vi "simulated image deformation.vi"(9 "Stop":bool, 11 "file path (use dialog)":path=path "F:/20240411-145056tdTomato zfluctuate dark small/20240411-145056tdTomato zfluctuate dark small.3DU16") -> ()   [LabVIEW 2024]
doc: "This example shows how to use the color pattern matching tools in NI Vision.\n\nYou use color pattern matching to locate known reference or fiducial patterns in an image quickly. Pattern matching is the key to many applications. Color pattern matching can provide your application with information about the presence or absence, number, and location of the model within an image.\n\nYou use color pattern matching in the following three general applications areas:\n\n* Alignment -- Determine the position and orientation of a known object by locating features. You use the features as points of reference on the object.\n\n* Gauging -- Measure lengths, diameters, angles, and other critical dimensions. If the measurements fall outside of set tolerance levels, the component is rejected. You sometimes use gauging in-line with the manufacturing process and off-line. If you make the measurements off-line, a sample of components is used to determine the quality of a lot or batch of manufactured components.\n\n* Inspection -- Detect simple flaws, such as missing parts or unreadable printing."
uses:
  <vilib>/gmath/NumericalOptimization/stopping criteria.ctl
  <vilib>/Analysis/baseanly.llb/Real A x B.vi
  <vilib>/Analysis/baseanly.llb/A x Vector.vi
  <vilib>/gmath/NumericalOptimization/Downhill Simplex.vi
  <vilib>/vision/NI_Vision_Development_Module.lvlib
  <vilib>/gmath/NI_Gmath.lvlib
  <vilib>/Analysis/NI_AALBase.lvlib
panel:
  in  "save transformed imgs":bool=TRUE
  out "A x B":dbl[][][](array[numeric])=[[[1.0252319039814008, 0.002391061207094415, -0.3573751785157772], [0.00737380006384733, 1.023351696337477, -5.931741689900512], [4.801742722373331e-05, -1.5076143397823732e-05, 1.0]], [[1.032657460981609, -0.004112535189805674, 0.9921109023203691], [0.014233192177529825, 1.0208690943004752, -7.9981262414118754], [7.030577164981777e-05, -4.3262018120171305e-05, 1.0001558400761408]], [[1.0416733185763245, 0.006155557532026288, -2.0796096172703544], [0.015025223132497195, 1.0275947891361181, -7.698789210595932], [9.848724819265994e-05, -4.749138408643344e-05, 1.0002152245800837]], [[1.055582542463075, 0.0225232241207663, -6.272162520913962], [0.015671378565617424, 1.0390878659055158, -6.578682702191399], [0.00011065087078061124, -1.1644079672646958e-05, 0.9999239310237085]], [[1.0696837271299575, 0.0504127718928557, -10.16158458953805], [0.016405251487257792, 1.0626775335818377, -6.853459701654355], [0.00012715279311096902, 5.854990616084134e-05, 0.9993898132887179]], [[1.0867852876742778, 0.05466443617762524, -10.645243835104656], [0.0215449194026129, 1.0885495889388574, -10.976399560961317], [0.00016645941245247426, 6.81093126769533e-05, 0.9989678064999458]], [[1.1109676198793976, 0.055385921129969956, -11.411221140746001], [0.02718487606984163, 1.1036287605452453, -13.550538925915514], [0.00021282122893302702, 6.923321844189429e-05, 0.9985256438980302]], [[1.1111042461542384, 0.050999241521229886, -10.754894691290525], [0.02730121211520052, 1.093865956251593, -12.65523517648029], [0.00022306723318648547, 3.6131640344551076e-05, 0.9988250940132484]], [[1.1118110959717575, 0.05618805365262508, -11.553002851896442], [0.027990916395066647, 1.0954167080541724, -11.28573727695852], [0.0002295058388808017, 4.6619913963022765e-05, 0.998647179090953]], [[1.1261894436159139, 0.09733031423529623, -19.260741205606603], [0.029220748081624653, 1.1165854803933235, -11.610522949858835], [0.00025346518882477767, 9.924433055073616e-05, 0.9978814999070178]]]
  out "Intensity Graph 7":dbl[][](graph)
  out "Intensity Graph 3":u16[][](graph)
  in  "z index":i32=48
  in  "quit review":bool
  in  "review index":i32=700
  out "Intensity Graph 2":u16[][](graph)
  out "Waveform Graph":dbl[][](graph)=[[0.0, -0.08806760786646446, -0.16032994108789017, -0.2183501586951051, -0.26369141971893734, -0.2979168831902148, -0.3225897081397656, -0.33927305359841764, -0.3495300785969989, -0.35492394216633755, -0.35701780333726146, -0.3573748211405988, -0.3328497292755918, -0.25364666922385326, -0.13116245216132086, 0.022798969999970276, 0.19643364534798619, 0.37793762197069186, 0.5555069479560524, 0.7173376713920336, 0.8516258403666004, 0.9465675029677187, 0.9903587072833533, 0.9650749491075363, 0.8574975473775769, 0.6782939355281823, 0.43882181480620885, 0.15043888645851322, -0.17549714826804919, -0.527628588126619, -0.8945977318703406, -1.2650468782523596, -1.6276183260258152, -1.9709543739438526, -2.296946156935724, -2.640927730904358, -3.0025556475511013, -3.3783195711163714, -3.7647091658405802, -4.158214095964146, -4.555324025727483, -4.952528619371011, -5.346317541135141, -5.733180455260291, -6.109607025986877, -6.48106926036093, -6.883860677888618, -7.311417492005393, -7.751127569084709, -8.190378775500008, -8.616558977624749, -9.017056041832381, -9.379257834496357, -9.690552221990131, -9.938327070687153, -10.109970246960875, -10.201151879841863, -10.267024567986702, -10.321911211707524, -10.367952569544704, -10.407289400038614, -10.44206246172963, -10.474412513158125, -10.506480312864474, -10.540406619389051, -10.57833219127223, -10.622397787054384, -10.675173119096588, -10.742515845409994, -10.822471601698131, -10.910905333332167, -11.003681985683269, -11.096666504122606, -11.185723834021344, -11.266718920750652, -11.335516709681697, -11.387982146185648, -11.419980175633668, -11.427288124583471, -11.405851457892762, -11.359375623120723, -11.293638889824585, -11.21441952756158, -11.127495805888934, -11.038645994363877, -10.953648362543642, -10.878281179985455, -10.818322716246547, -10.779551240884148, -10.767640545611597, -10.776910242635998, -10.800863446106137, -10.838842296024412, -10.89018893239322, -10.954245495214964, -11.030354124492039, -11.117856960226845], [0.0, -0.6990844119063075, -1.377904026033752, -2.0323701215933294, -2.658393977796034, -3.251886873852863, -3.808760088974812, -4.324924902372875, -4.79629259325805, -5.21877444084133, -5.588281724333714, -5.900725722946196, -6.176724297406029, -6.449291732458249, -6.714149880756897, -6.9666333680901396, -7.202076820246148, -7.415814863013091, -7.603182122179137, -7.759513223532458, -7.880142792861221, -7.960405455953598, -7.995635838597756, -7.9948336322923925, -7.986480781535741, -7.972204257323417, -7.952558476324648, -7.928097855208662, -7.899376810644687, -7.86694975930195, -7.83137111784968, -7.793195302957104, -7.75297673129345, -7.711269819527946, -7.660478807106392, -7.5779837528866185, -7.469326611741255, -7.342219431575375, -7.2043742602940535, -7.0635031458023665, -6.927318136005389, -6.803531278808196, -6.699854622115862, -6.624000213833463, -6.583680101866072, -6.579962872361264, -6.585233956995526, -6.595346634978383, -6.610147040936223, -6.629481309495433, -6.6531955752824, -6.681135972923512, -6.713148637045156, -6.749079702273719, -6.788775303235589, -6.832081574557153, -6.891291945954723, -7.053502480097667, -7.3192333957798015, -7.668537856253234, -8.081469024770076, -8.538080064582442, -9.01842413894243, -9.502554411102155, -9.970524044313727, -10.402386201829254, -10.778194046900845, -11.084284209007102, -11.385729309992561, -11.698136370665495, -12.012812146340236, -12.32106339233112, -12.614196863952477, -12.883519316518646, -13.120337505343956, -13.31595818574274, -13.46168811302933, -13.548834042518063, -13.569906497288047, -13.551957342469379, -13.51166631084667, -13.452158545978971, -13.376559191425343, -13.287993390744841, -13.18958628749652, -13.084463025239433, -12.975748747532641, -12.866568597935194, -12.760047720006153, -12.659065885842333, -12.543790814013336, -12.40520389539235, -12.250530202818402, -12.086994809130518, -11.921822787167729, -11.762239209769062, -11.61546914977354], [498.0, 498.05959291224764, 498.1109505097321, 498.1546182800102, 498.19114171063876, 498.22106628917453, 498.2449375031743, 498.2633008401948, 498.27670178779294, 498.2856858335255, 498.2907984649492, 498.29258516962085, 498.28854436784206, 498.27453904241014, 498.2509591731421, 498.2182421278122, 498.1768252741945, 498.1271459800634, 498.0696416131931, 498.00474954135774, 497.93290713233154, 497.85455175388876, 497.7701207738036, 497.61713712408425, 497.2777173834449, 496.78789154147364, 496.1891634558678, 495.52303698432473, 494.8310159845418, 494.1546043142164, 493.53530583104583, 493.01462439272746, 492.6340638569586, 492.4351280814367, 492.4055259436575, 492.392373253152, 492.38226987404346, 492.3744822410049, 492.3682767887094, 492.3629199518301, 492.3576781650401, 492.3518178630124, 492.34460548042017, 492.3353074519365, 492.3231902122344, 492.30650694071056, 492.28031112090554, 492.2448781840679, 492.2011884696724, 492.1502223171939, 492.0929600661073, 492.0303820558875, 491.9634686260093, 491.8932001159475, 491.820556865177, 491.74651921317275, 491.66865653803535, 491.5644471740417, 491.43579776771617, 491.29028385163474, 491.1354809583733, 490.9789646205077, 490.82831037061396, 490.69109374126793, 490.57489026504555, 490.4872754745227, 490.4358249022752, 490.4257655490913, 490.43149698256036, 490.44293482140483, 490.458727548562, 490.4775236469694, 490.49797159956444, 490.51871988928445, 490.5384169990669, 490.5557114118492, 490.56925161056876, 490.577686078163, 490.57847624470804, 490.5401514953157, 490.4548658284808, 490.33021692570134, 490.1738024684751, 489.99322013829993, 489.7960676166738, 489.5899425850944, 489.38244272505966, 489.18116571806746, 488.99370924561566, 488.8275830414089, 488.67949517238, 488.54146103744847, 488.4096151399728, 488.2800919833113, 488.14902607082234, 488.01255190586426, 487.8668039917954], [0.0, -0.34659355840331935, -0.6697552209281179, -0.967562437605149, -1.2380926584651664, -1.4794233335389235, -1.689631912857174, -1.8667958464506709, -2.0089925843501684, -2.1142995765864194, -2.1807942731901786, -2.2065541241921984, -2.187944773997436, -2.1261760296745087, -2.0289093348903626, -1.9038526962348445, -1.7587141202978014, -1.6012016136690805, -1.439023182938529, -1.2798868346959935, -1.1315005755313214, -1.0015724120343592, -0.8978103507949546, -0.8196809058998543, -0.7514634450780548, -0.690599285840092, -0.6351229030496413, -0.5830687715703788, -0.5324713662659806, -0.4813651620001232, -0.4277846336364825, -0.3697642560387343, -0.3053385040705554, -0.23254185259562143, -0.14456043497485793, -0.027999389199703073, 0.11114401645705166, 0.2654873174264595, 0.42764804913957155, 0.590243747027441, 0.7458919465211207, 0.8872101830516632, 1.0068159920501203, 1.097326908947545, 1.1513604691749901, 1.1688676165503586, 1.180922417594905, 1.191940545301066, 1.2018861553343343, 1.210723403360202, 1.2184164450441612, 1.224929436051705, 1.230226532048325, 1.2342718886995137, 1.2370296616707637, 1.2384640066275672, 1.231821935776551, 1.170744324711977, 1.0569070651791723, 0.9031435851839223, 0.7222873127320133, 0.5271716758292289, 0.33063010248135905, 0.14549602069418777, -0.015397141526498848, -0.1392159561749151, -0.213126995245275, -0.22806519538413308, -0.22410185444698455, -0.2157144573525903, -0.20328602675556465, -0.187199585310522, -0.16783815567207672, -0.1455847604948432, -0.12082242243343559, -0.09393416414246869, -0.06530300827655669, -0.03531197749031392, -0.004049634139276918, 0.0359271098690905, 0.0871275237671033, 0.14837358367929487, 0.21848726573019667, 0.2962905460443419, 0.3806054007462635, 0.47025380596049393, 0.5640577378115662, 0.6608391724240136, 0.7594200859223673, 0.8588240958035979, 0.976263368252154, 1.1185316498879931, 1.2787694647325516, 1.4501173368072657, 1.625715790133572, 1.798705348732907, 1.96222653662671], [498.0, 498.352995504663, 498.6963739058205, 499.0290531199109, 499.3499510633724, 499.65798565264345, 499.9520748041623, 500.23113643436733, 500.49408845969685, 500.7398487965893, 500.96733536148287, 501.17546607081596, 501.37464179085134, 501.5789093950214, 501.7835485008412, 501.98365143314686, 502.1743105167747, 502.35061807656086, 502.50766643734164, 502.6405479239532, 502.74435486123184, 502.81417957401374, 502.8451143871352, 502.82378743572696, 502.7356884268529, 502.5925893443046, 502.4070972806018, 502.1918193282643, 501.9593625798119, 501.7223341277643, 501.49334106464136, 501.2849904829628, 501.10988947524845, 500.98064513401806, 500.8987728782318, 500.8335975692704, 500.77961668207456, 500.7338112382921, 500.6931622595708, 500.65465076755834, 500.6152577839025, 500.5719643302511, 500.5217514282519, 500.4616000995526, 500.38849136580103, 500.2921931047241, 500.1402738909532, 499.93828511817765, 499.69684350399683, 499.42656576601024, 499.13806862181735, 498.84196878901764, 498.5488829852105, 498.2694279279956, 498.01422033497215, 497.7938769237398, 497.61279826542494, 497.4325400401901, 497.24841032488905, 497.06512645930275, 496.887405783212, 496.7199656363976, 496.56752335864036, 496.43479628972113, 496.32650176942064, 496.2473571375198, 496.20207973379945, 496.19311773343514, 496.1942811140667, 496.19680986244845, 496.2006685681868, 496.20582182088845, 496.2122342101597, 496.2198703256072, 496.2286947568374, 496.2386720934568, 496.2497669250719, 496.2619438412893, 496.27675996106404, 496.3345542190964, 496.4438852365347, 496.5925793326237, 496.76846282660824, 496.9593620377332, 497.15310328524333, 497.33751288838346, 497.50041716639845, 497.62964243853304, 497.71301502403213, 497.73842217131727, 497.70385651449106, 497.61900493959655, 497.49237882358017, 497.3324895433883, 497.1478484759674, 496.9469669982638, 496.738356487224], [299.0, 298.8687898245559, 298.74114208501135, 298.61822224462526, 298.5011957666566, 298.3912281143645, 298.2894847510077, 298.19713113984534, 298.11533274413637, 298.0452550271398, 297.98806345211443, 297.94492348231944, 297.9134972964784, 297.88817502359996, 297.86760770201903, 297.85049603737355, 297.8355407353016, 297.82144250144114, 297.80690204143025, 297.7906200609068, 297.77129726550896, 297.7476343608746, 297.7183320526418, 297.6729729654948, 297.5946975659272, 297.49035444654606, 297.3676103274553, 297.23413192875864, 297.0975859705601, 296.9656391729634, 296.84595825607255, 296.74620993999133, 296.6740609448236, 296.6371779906733, 296.63285238579186, 296.6314376949938, 296.6303894838692, 296.6296134483004, 296.6290152841698, 296.6285006873597, 296.6279753537525, 296.6273449792306, 296.62651525967635, 296.6253918909721, 296.62388056900016, 296.6140899421671, 296.5617806883245, 296.47048352115365, 296.3490125456797, 296.20618186692786, 296.0508055899233, 295.8916978196913, 295.7376726612569, 295.5975442196455, 295.4801265998821, 295.3942339069921, 295.3449895176176, 295.3096259667366, 295.28117834008566, 295.2579055224981, 295.23806639880723, 295.21991985384636, 295.20172477244876, 295.18174003944773, 295.15822453967667, 295.12943715796877, 295.0936367791574, 295.04652465511975, 294.9565215236572, 294.82231536714386, 294.6536774701274, 294.4603791171553, 294.2521915927753, 294.0388861815351, 293.8302341679821, 293.6360068366641, 293.4659754721286, 293.32991135892325, 293.2363100581014, 293.15805098242436, 293.0815909138026, 293.0081523302429, 292.9389577097521, 292.8752295303369, 292.81819027000427, 292.76906240676084, 292.72906841861345, 292.69943078356897, 292.6813719796341, 292.6761269685125, 292.6852826941717, 292.70728856110696, 292.7392532875312, 292.77828559165727, 292.8214941916981, 292.8659878058665, 292.9088751523754], [0.0, 0.07070781292600659, 0.13222535643952152, 0.18507884903170793, 0.22979450919372876, 0.2668985554167473, 0.2969172061919265, 0.32037668001042946, 0.33780319536341913, 0.3497229707420588, 0.3566622246375115, 0.35914717554094033, 0.3482915577971586, 0.3131532160574969, 0.2588059350305878, 0.19048024915228876, 0.11340669285845648, 0.03281580058494821, -0.04606189323237858, -0.11799585415766728, -0.1777555477550603, -0.22011043958870102, -0.23982999522273174, -0.24086489926704457, -0.24116329701618808, -0.2414315752675673, -0.24166968279406276, -0.241877568368555, -0.24205518076392457, -0.24220246875305196, -0.24231938110881773, -0.2424058666041024, -0.2424618740117865, -0.24248735210475061, -0.23928013016051664, -0.22283171328184445, -0.19318622311013947, -0.15120424894823825, -0.0977463800989781, -0.03367320586519559, 0.0401546844502724, 0.12287670154458954, 0.21363225611491807, 0.3115607588584216, 0.4158016204722639, 0.5473850940108563, 0.8007768483608195, 1.1636471126890497, 1.6087885959256754, 2.10899400700081, 2.637056054844583, 3.1657674483871165, 3.6679208965585346, 4.11630910828896, 4.483724792508517, 4.7429606581473305, 4.881562758598475, 4.993013262607376, 5.098027226909434, 5.19561631939748, 5.284792207964345, 5.364566560502858, 5.433951044905852, 5.491957329066154, 5.537597080876598, 5.569881968230012, 5.587823659019229, 5.59039759879764, 5.577098493956473, 5.549774150877927, 5.510655747529718, 5.461974461879563, 5.405961471895177, 5.344847955544278, 5.280865090794581, 5.216244055613805, 5.153216027969664, 5.094012185829876, 5.040405899432335, 4.982287519870069, 4.916765597399062, 4.846611267084489, 4.774595663991526, 4.703489923185351, 4.636065179731137, 4.575092568694061, 4.5233432251393, 4.483588284132028, 4.458598880737424, 4.451115797259061, 4.460208131096691, 4.48350644105839, 4.5200988580289145, 4.569073512893016, 4.629518536535451, 4.700522059840971, 4.781172213694331], [299.0, 299.33625940798174, 299.66277170316766, 299.9749671330503, 300.2682759451221, 300.53812838687554, 300.7799547058031, 300.9891851493973, 301.16124996515055, 301.2915794005554, 301.3756037031043, 301.40875312028965, 301.4032885902406, 301.38452928812944, 301.35551881264746, 301.3190529383504, 301.27792743979387, 301.23493809153354, 301.19288066812516, 301.1545509441243, 301.12274469408663, 301.1002576925679, 301.08988571412374, 301.1191111280352, 301.23592110019075, 301.4268187584476, 301.6761400658353, 301.9682209853833, 302.28739748012123, 302.6180055130785, 302.94438104728476, 303.2508600457695, 303.5217784715623, 303.74147228769255, 303.91007911393206, 304.07017478948, 304.2246408140779, 304.3726836529518, 304.51350977132813, 304.646325634433, 304.7703377074927, 304.88475245573335, 304.9887763443812, 305.0816158386626, 305.16247740380356, 305.23059918879653, 305.28671703298335, 305.33335733023785, 305.3731385253697, 305.40867906318846, 305.44259738850366, 305.47751194612493, 305.51604118086186, 305.56080353752395, 305.61441746092095, 305.67950139586225, 305.76394374671406, 305.9055807461334, 306.10261825323084, 306.3443419748811, 306.6200376179591, 306.91899088933945, 307.23048749589714, 307.5438131445068, 307.8482535420433, 308.1330943953814, 308.3876214113959, 308.60380113913635, 308.8085558196718, 309.01059948458266, 309.20861919323085, 309.4013020049782, 309.5873349791867, 309.7654051752182, 309.9341996524345, 310.09240547019755, 310.2387096878693, 310.3717993648115, 310.4905008780819, 310.59795116076054, 310.696903954187, 310.7886709848619, 310.8745639792859, 310.9558946639597, 311.033974765384, 311.11011601005947, 311.1856301244868, 311.2618288351666, 311.3400238685996, 311.42147856390994, 311.5027067532546, 311.58148314562163, 311.6586124780547, 311.7348994875973, 311.811148911293, 311.8881654861853, 311.9667539493179]]
  in  "stop":bool
  in  "skip matching":bool
  out "size(s)":i32[](array[numeric])=[159, 184]
  out "transform index":i32=998
  out "error out 2":errorcluster
  out "error out":errorcluster
  in  "mabiki":i32=10
  out "appended array 3":i32[](array[numeric])=[184, 159]
  out "minimum 2":dbl[](array[numeric])=[49.34280549447182, 30.507003653054642, 447.31274204038084, 30.457516913102424, 447.59510849908503, 269.39846570126116, 53.656175912030534, 269.1288380732932]
  out "appended array 2":sgl[](array[numeric])
  out "appended array":dbl[](array[numeric])=[50.0, 30.0, 449.0, 270.0]
  out "Numeric":i32=9993
  out "num of volumes":i32=9995
  out "sqrt(x) 4":dbl=2040.3038989327056
  out "sqrt(x) 3":dbl
  out "sqrt(x) 2":dbl=910.3411448462604
  out "sqrt(x)":dbl=891.563233876319
  out "max value 2":dbl=16649.0
  out "max value":dbl=16161.0
  out "minimum":dbl[](array[numeric])=[155.64411652807632, 68.43640121785279, 338.3202861949042, 68.35157731671751, 340.3174931085275, 225.28530291703504, 161.01996406448592, 233.55726960411664]
  out "number of function evaluations":i32=252
  out "f(minimum)":dbl=794885.0 format="%#_6f"
  out "Global Rectangle":i32[](array[numeric])=[156, 71, 340, 230]
  out "Intensity Graph 6":i16[][](graph)
  in  "stopping criteria":T1={"function tolerance"=100.0, "parameter tolerance"=0.0001, "max iterations"=2000, "max function calls"=100000, "gradient tolerance"=1e-06, "max time (sec)"=-1.0}
  in  "y":i32=5
  in  "max 3":dbl=100.0
  out "Intensity Graph 5":i16[][](graph)
  out "Matches (pixel)":T2(array[cluster])=[{"Position"={"x"=247.77678, "y"=146.75125}, "Angle"=0.9103387, "Scale"=1.0, "Score"=963.9151, "Bounding Box"=[{"x"=155.0332, "y"=69.21496}, {"x"=338.0101, "y"=66.30749}, {"x"=340.52036, "y"=224.28754}, {"x"=157.54346, "y"=227.195}, {"x"=155.0332, "y"=69.21496}]}] {"Bounding Box"."y" format="%.2f"; "Bounding Box"."x" format="%.2f"; "Score" format="%.2f"; "Scale" format="%.2f"; "Angle" format="%.2f"; "Position"."y" format="%.2f"; "Position"."x" format="%.2f"}
  out "ROI":T3={"Global Rectangle"=[156, 71, 340, 230], "Contours"=[{"Contour Type"=0, "ROI Type"=3, "Points"=[156, 71, 340, 230]}]}
  out "Image 2":T4(plugin-control)
  in  "z pos":i32=87
  in  "volume":i32=458
  in  "channel":i32
  in  "proj/slice":bool=TRUE
  in  "min":dbl
  in  "max":dbl=1.0
  in  "Array 2":u32[](array[colorbox])=[0, 16711680, 16776960, 16448250, 16776960, 16711680, 16448250, 16448250]
  in  "num of colors":i32=4
  in  "zoom":dbl=0.600000000000001 format="%_2g"
  out "Intensity Graph":dbl[][](graph)
  out "dimensions \n(vol, ch, z, y, x)":i32[](array[numeric])=[9995, 2, 97, 300, 499]
  out "voxel size \n(z, y, x)":dbl[](array[numeric])=[0.4095, 0.4095, 0.4095]
  out "Number of Matches":i32=1
  in  "Max # of Matches":i32=1
  in  "Minimum Score":sgl=800.0
  out "Image":T4(plugin-control)
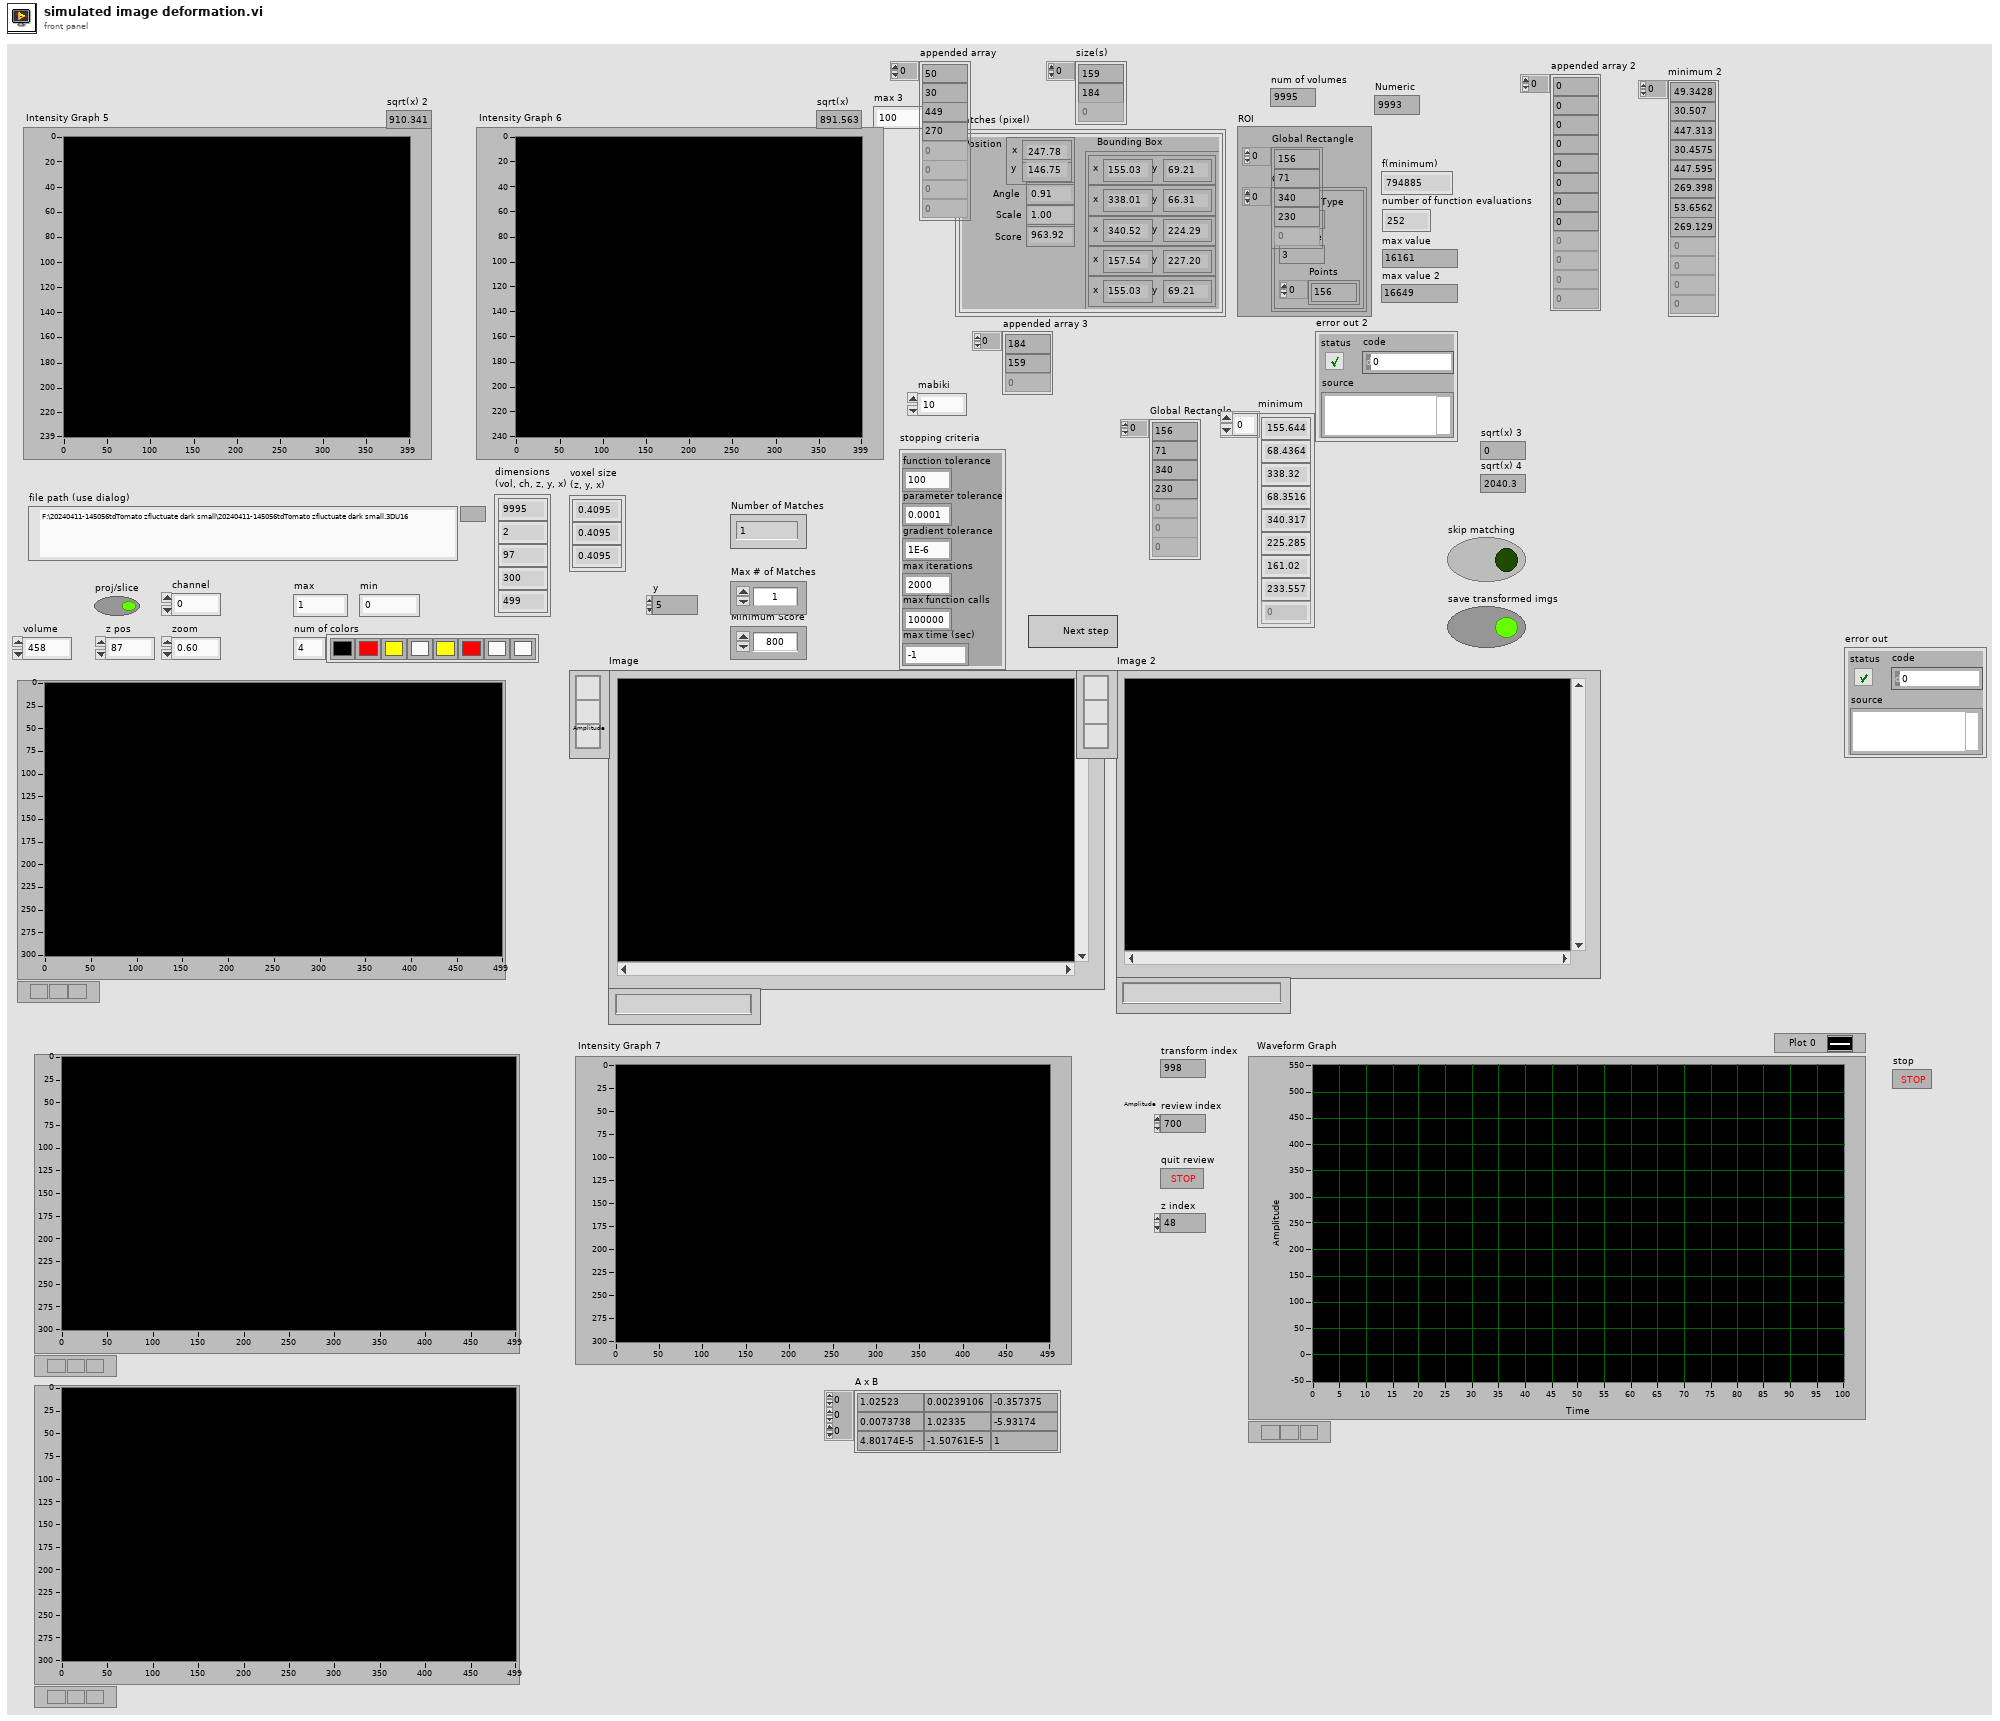
[diagram p1: front panel]
types:
  T1 = typedef "NI_Gmath.lvlib/stopping criteria.ctl" = cluster{"function tolerance":dbl, "parameter tolerance":dbl, "max iterations":i32, "max function calls":i32, "gradient tolerance":dbl, "max time (sec)":dbl}
  T2 = cluster{"Position":cluster{"x":sgl, "y":sgl}, "Angle":sgl, "Scale":sgl, "Score":sgl, "Bounding Box":cluster{"x":sgl, "y":sgl}[]}[]
  T3 = cluster{"Global Rectangle":i32[], "Contours":cluster{"Contour Type":u32, "ROI Type":u32, "Points":i32[]}[]}
  T4 = typedef "IMAQ Image.ctl" = refnum<image>
  T5 = enum16{"open", "replace", "create", "open or create", "replace or create", "replace or create with confirmation"}
  T6 = typedef "Image Type" = u32
  T7 = typedef "IMAQ Rectangle" = cluster{"Left":i32, "Top":i32, "Right":i32, "Bottom":i32, "Rotation":dbl}
  T8 = typedef "ROI Descriptor" = cluster{"Global Rectangle":i32[], "Contours":cluster{"ID":enum32{"External", "Internal"}, "Type":u32, "Coordinates":i32[]}[]}
  T9 = cluster{"Interpolation Type":enum32{"Zero Order", "Bilinear", "Quadratic", "Cubic", "Bilinear Fixed"}, "Destination Width":u32, "Destination Height":u32, "Fill Value":sgl}
  T10 = cluster{"template":u8[][], "target img":u8[][], "image size":dbl[]}
  T11 = cluster{"Max # of Matches":i32, "Minimum Score":sgl}
  T12 = cluster{"Max # of Matches":i32, "Minimum Score":sgl, "Angle Ranges":cluster{"Start Angle":sgl, "End Angle":sgl}[]}
  T13 = cluster{"Position":cluster{"x":sgl, "y":sgl}, "Angle":sgl, "Scale":sgl, "Score":sgl, "Bounding Box":cluster{"x":sgl, "y":sgl}[]}
  T14 = cluster{i32[], cluster{"Contour Type":u32, "ROI Type":u32, i32[]}[]}
  T15 = cluster{"output tetragon rigid":dbl[][], "output tetragon proj":dbl[][], "error rigid":dbl[], "error proj":dbl[], "input rectangle":dbl[], "image size":dbl[]}
  T16 = typedef "NI_Matrix.lvlib/RealMatrix.ctl" = dbl[][]
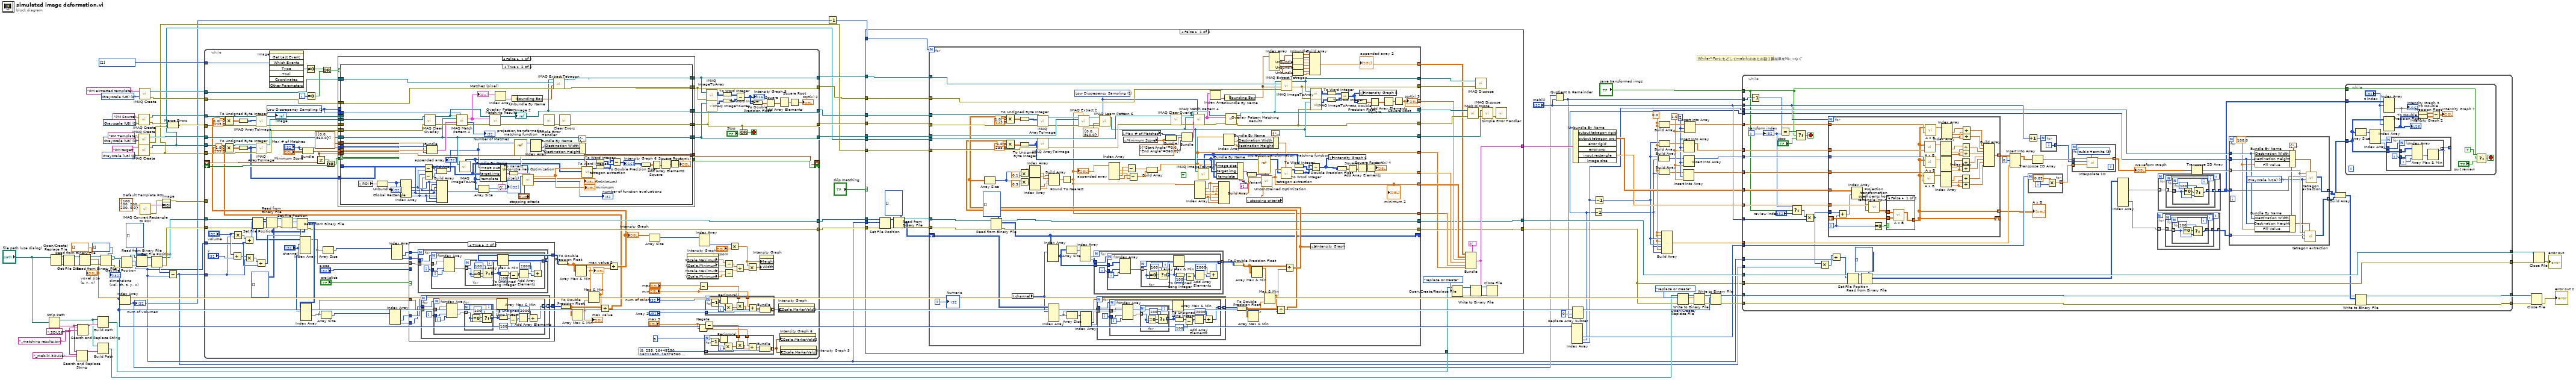
[diagram p0: block diagram]
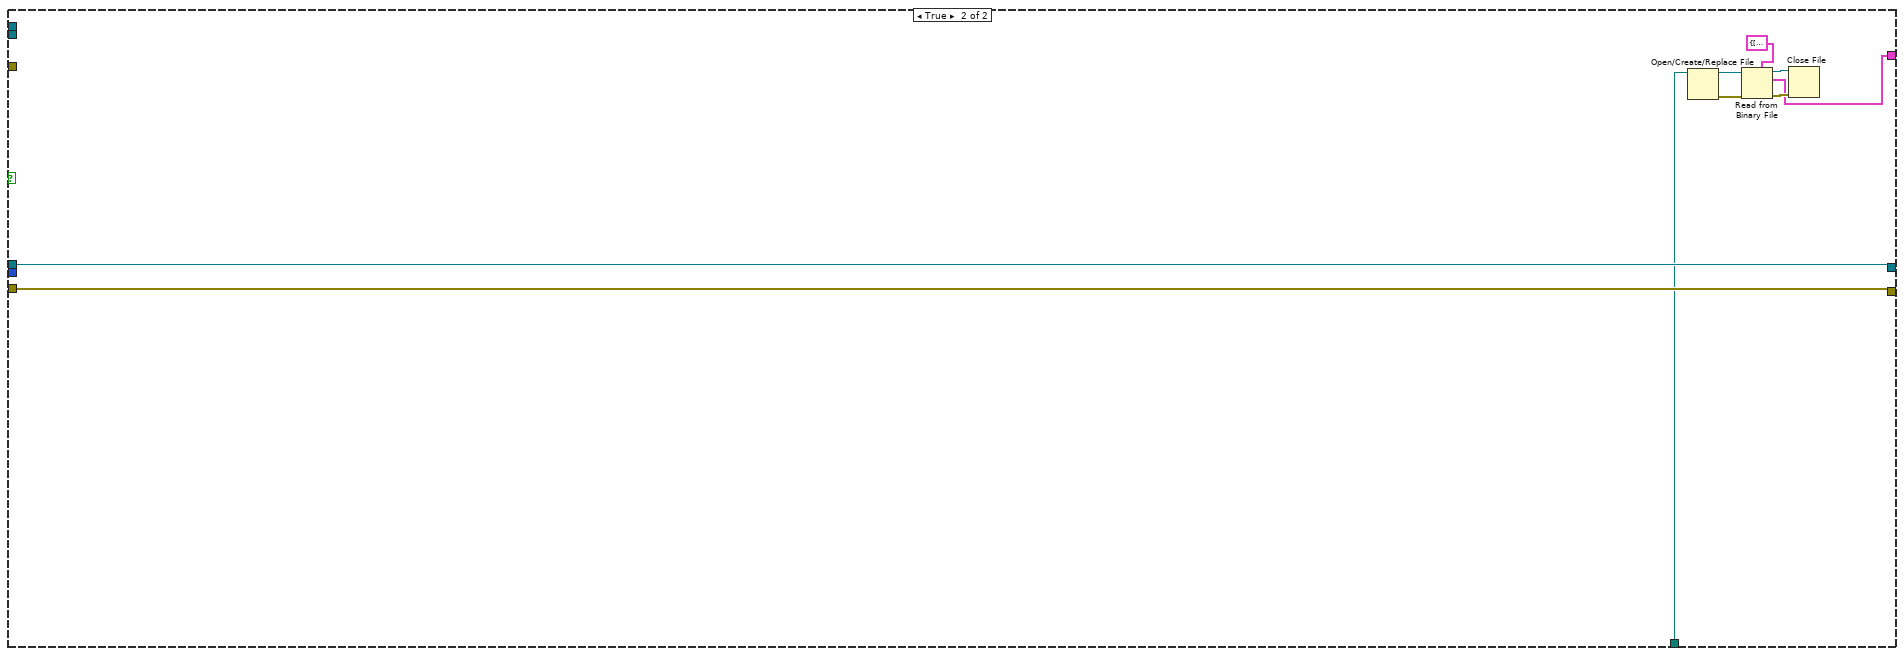
[diagram p3: hidden frame]
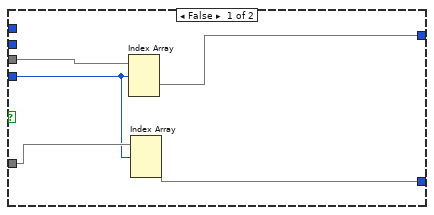
[diagram p4: hidden frame]
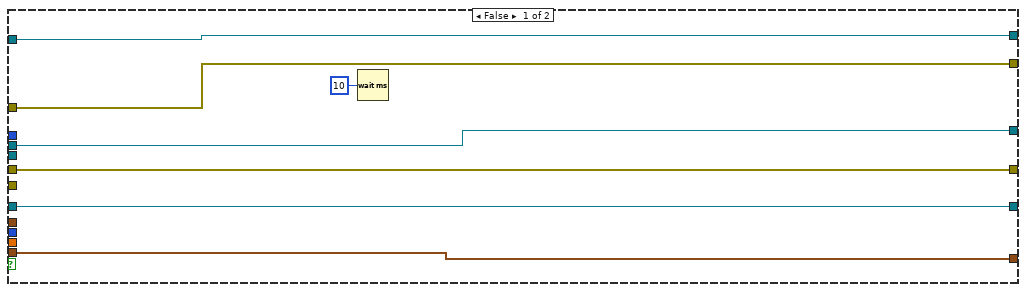
[diagram p5: hidden frame]
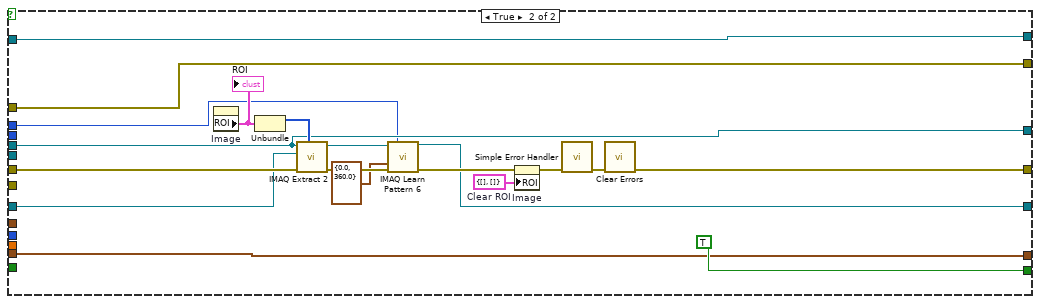
[diagram p6: hidden frame]
diagram:
  w21 = ".3DU16" ("search string")
  w54 = 1.0 ("new element/subarray")
  w53 = 2 ("index")
  w45 = 0.0 ("element")
  w70 = T6 0 items=["Grayscale (U8)", "Grayscale (I16)", "Grayscale (SGL)", "Complex (CSG)", "RGB (U32)", "HSL (U32)", "RGB (U64)", "Grayscale (U16)"] ("Image Type")
  w72 = T6 0 items=["Grayscale (U8)", "Grayscale (I16)", "Grayscale (SGL)", "Complex (CSG)", "RGB (U32)", "HSL (U32)", "RGB (U64)", "Grayscale (U16)"] ("Image Type")
  w98 = T6 0 items=["Grayscale (U8)", "Grayscale (I16)", "Grayscale (SGL)", "Complex (CSG)", "RGB (U32)", "HSL (U32)", "RGB (U64)", "Grayscale (U16)"] ("Image Type")
  w99 = T6 0 items=["Grayscale (U8)", "Grayscale (I16)", "Grayscale (SGL)", "Complex (CSG)", "RGB (U32)", "HSL (U32)", "RGB (U64)", "Grayscale (U16)"] ("Image Type")
  w101 = i32[] [2] items=["No Event"=0, "Click Event"=1, "Draw Event"=2, "Size Event"=4, "Scroll Event"=5, "Double Click Event"=8] ("Which Events")
  w102 = T7 {"Left"=100, "Top"=100, "Right"=200, "Bottom"=200, "Rotation"=0.0}  # Default Template ROI
  # "While->Forにもどしてmabikiのあとの割り算結果をNにつなぐ"
  n1 = Strip Path(path="file path (use dialog)") -> (stripped path=w20:path, name=w22:string)
  n2 = Open/Create/Replace File(file path (use dialog)="file path (use dialog)") -> (refnum out=w91:refnum<file>, error out=w92:errorcluster)  [unwired: 5 in, 1 out]
  n3 = Get File Size(file=w91, error in=w92) -> (refnum out=w90:refnum<file>, 0:w89:errorcluster)  [unwired: 1 out]
  n4 = Search and Replace String(input string=w22, search string=w21, replace string="_mabiki.3DU16") -> (result string=w19:string)  [unwired: 5 in, 3 out]
  n5 = Search and Replace String(input string=w22, search string=w21, replace string="_matching results.bin") -> (result string=w34:string)  [unwired: 5 in, 3 out]
  n6 = Read from Binary File(5:dbl[] [] ("voxel size [um]"), 8:w89, 11:w90) -> (0:w87:errorcluster, 2:w17:dbl[], 3:w88:refnum<file>)  [unwired: 3 in, 1 out]
  "voxel size \n(z, y, x)" <- w17
  n7 = Build Path(base path=w20, name or relative path=w34) -> (appended path=w56:path)
  n8 = Build Path(base path=w20, name or relative path=w19) -> (appended path=w18:path)
  n9 = Read from Binary File(5:i32[] [] ("voxel number"), 8:w87, 11:w88) -> (0:w84:errorcluster, 2:w14:i32[], 3:w83:refnum<file>)  [unwired: 3 in, 1 out]
  "dimensions \n(vol, ch, z, y, x)" <- w14
  n10 = Index Array(array=w14) -> (element=w13:i32)  [unwired: 1 in]
  "num of volumes" <- w13
  n11 = Get File Position(4:w84, 7:w83) -> (0:w76:errorcluster, 2:w11:i64, 3:w75:refnum<file>)
  n12 = Read from Binary File(5:u16[][][][] [], 8:w76, 11:w75) -> (0:w80:errorcluster, 3:w79:refnum<file>)  [unwired: 3 in, 2 out]
  n13 = call "IMAQ Create"("Image Name"="PM Template", "Image Type"=w98) -> ("New Image"=w100:T4, "error out"=w96:errorcluster)  [unwired: 3 in]
  n14 = call "IMAQ Create"("Image Name"="PM target", "Image Type"=w72) -> ("New Image"=w61:T4, "error out"=w60:errorcluster)  [unwired: 3 in]
  n15 = call "IMAQ Create"("Image Name"="PM Source", "Image Type"=w99) -> ("New Image"=w82:T4, "error out"=w81:errorcluster)  [unwired: 3 in]
  n16 = call "IMAQ Create"("Image Name"="PM extracted template", "Image Type"=w70) -> ("New Image"=w68:T4, "error out"=w67:errorcluster)  [unwired: 3 in]
  n17 = call "IMAQ Convert Rectangle to ROI"("Rectangle"=w102) -> ("error out"=w97:errorcluster, "ROI Descriptor"=w94:T8)  [unwired: 8 in]
  n18 = Get File Position(4:w80, 7:w79) -> (0:w74:errorcluster, 2:w78:i64, 3:w73:refnum<file>)
  n19 = property on="Image" class="ImageControl"(error in=w97, "ROI"=w94) -> (error out=w93:errorcluster)  [unwired: 1 in, 1 out]
  n20 = Merge Errors(w81, w96) -> (w95:errorcluster)
  n21 = Subtract(x=w78, y=w11) -> (x-y=w10:i64)
  n22 = while {
    tunnel: w82 -> [w157]
    tunnel: w101 -> [w222]
    tunnel: w100 -> [w213]
    tunnel: w95 -> [w156]
    shift-right: [w212] -> _
    shift-left: _ -> [w208]
    shift-right: [w216] -> _
    shift-left: _ -> [w215]
    tunnel: [w135] -> w64
    tunnel: [w124] -> w62
    tunnel: [w134] -> w63
    tunnel: w93 -> [_]
    tunnel: w11 -> [w161]
    tunnel: [w160] -> w58
    tunnel: [w159] -> w59
    tunnel: w10 -> [w154]
    tunnel: w74 -> [w153]
    tunnel: w73 -> [w152]
    tunnel: w61 -> [w144]
    tunnel: w60 -> [w141]
    tunnel: w68 -> [w139]
    tunnel: w67 -> [w138]
    tunnel: [w137] -> w66
    tunnel: [w136] -> w65
    i -> [w219]
    stop <- w205 stop-if-true
    w114 = 1 items=["All", "Low Discrepancy Sampling", "Grayscale Value Pyramid", "Gradients Pyramid"] ("Algorithm")
    w163 = u16[][][][] []
    n23 = Add(x="volume", y="y") -> (x+y=w197:i32)
    n24 = Multiply(x="volume", y=w154) -> (x*y=w189:i64)
    n25 = Add(x=w189, y=w161) -> (x+y=w191:i64)
    n26 = Multiply(x=w197, y=w154) -> (x*y=w196:i64)
    n27 = Set File Position(offset (in bytes) (0)=w191, refnum=w152, error in=w153) -> (refnum out=w187:refnum<file>, error out=w188:errorcluster)  [unwired: 1 in]
    n28 = Add(x=w196, y=w161) -> (x+y=w198:i64)
    n29 = Read from Binary File(5:w163, 8:w188, 11:w187) -> (0:w105:errorcluster, 2:w190:u16[][][][], 3:w106:refnum<file>)  [unwired: 3 in, 1 out]
    n30 = invoke on="Image" class="ImageControl" method="Get Last Event"("Which Events"=w222) -> ("Type"=w221:i32)  [unwired: 7 in, 7 out]
    n31 = Set File Position(offset (in bytes) (0)=w198, refnum=w106, error in=w105) -> (refnum out=w193:refnum<file>, error out=w194:errorcluster)  [unwired: 1 in]
    n32 = Read from Binary File(5:w163, 8:w194, 11:w193) -> (0:w160:errorcluster, 2:w203:u16[][][][], 3:w159:refnum<file>)  [unwired: 3 in, 1 out]
    n33 = Index Array(array=w190, index (dim 0)="channel") -> (element=w186:u16[][][])  [unwired: 3 in]
    n34 = Index Array(array=w203, index (dim 0)="channel") -> (element=w204:u16[][][])  [unwired: 3 in]
    n35 = Bundle("Max # of Matches"="Max # of Matches", "Minimum Score"="Minimum Score") -> (w209:T11)  [unwired: 1 in]
    n36 = Not Equal To 0?(x=w221) -> (x != 0?=w220:bool)
    n37 = Equal To 0?(x=w219) -> (x = 0?=w218:bool)
    n38 = Not Equal?(x=w209, y=w208) -> (x != y?=w207:bool)
    n39 = Array Size(array=w204) -> (size(s)=w199:i32[])
    n40 = Or(x=w220, y=w218) -> (x .or. y?=w217:bool)
    n41 = Array Size(array=w186) -> (size(s)=w182:i32[])
    n42 = Or(x=w207, y=w215) -> (x .or. y?=w214:bool)
    n43 = Index Array(array=w199) -> (element #2=w201:i32, element #3=w202:i32)  [unwired: 3 in, 1 out]
    n44 = Index Array(array=w182) -> (element #2=w183:i32, element #3=w184:i32)  [unwired: 3 in, 1 out]
    n45 = case shown="True" "proj/slice" {
      tunnel: w183 -> [_ w246]
      tunnel: w184 -> [_ w245]
      tunnel: [w237 w244] -> w123
      tunnel: w186 -> [w238 w243]
      tunnel: "z pos" -> [w234 _]
      tunnel: w201 -> [_ w242]
      tunnel: w202 -> [_ w241]
      tunnel: w204 -> [w236 w240]
      tunnel: [w235 w239] -> w122
      frame False {
        n46 = Index Array(array=w238, index (dim 0)=w234) -> (element=w237:u16[][])  [unwired: 2 in]
        n47 = Index Array(array=w236, index (dim 0)=w234) -> (element=w235:u16[][])  [unwired: 2 in]
      }
      frame True {
        n48 = for {
          N: w246 -> [_]
          tunnel: w243 -> [w269]
          tunnel: [w267] -> w244 mode=indexing
          tunnel: w245 -> [w266]
          i -> [w268]
          n49 = for {
            N: w266 -> [_]
            tunnel: w269 -> [w280]
            tunnel: w268 -> [w279]
            tunnel: [w270] -> w267 mode=indexing
            i -> [w278]
            n50 = Index Array(array=w280, index (dim 1)=w279, index (dim 2)=w278) -> (element=w272:u16[])  [unwired: 1 in]
            n51 = for {
              tunnel: w272 -> [w283] mode=indexing
              tunnel: [w281] -> w271 mode=indexing
              n52 = Equal To 0?(x=w283) -> (x = 0?=w284:bool)
              n53 = Select(t=u16 100, s=w284, f=w283) -> (s? t:f=w281:u16)
            }
            n54 = Array Max & Min(array=w271) -> ()  [unwired: 4 out]
            n55 = To Unsigned Long Integer(number=w271) -> (unsigned 32bit integer=w277:u32[])
            n56 = Subtract(x=w277, y=100) -> (x-y=w276:u32[])
            n57 = Add Array Elements(numeric array=w276) -> (sum=w275:u32)
            n58 = Add(x=u32 2000, y=w275) -> (x+y=w270:u32)
          }
        }
        n59 = for {
          N: w242 -> [_]
          tunnel: w240 -> [w250]
          tunnel: w241 -> [w248]
          tunnel: [w247] -> w239 mode=indexing
          i -> [w249]
          n60 = for {
            N: w248 -> [_]
            tunnel: w250 -> [w261]
            tunnel: w249 -> [w260]
            tunnel: [w251] -> w247 mode=indexing
            i -> [w259]
            n61 = Index Array(array=w261, index (dim 1)=w260, index (dim 2)=w259) -> (element=w252:u16[])  [unwired: 1 in]
            n62 = for {
              tunnel: w252 -> [w264] mode=indexing
              tunnel: [w262] -> w253 mode=indexing
              n63 = Equal To 0?(x=w264) -> (x = 0?=w265:bool)
              n64 = Select(t=u16 100, s=w265, f=w264) -> (s? t:f=w262:u16)
            }
            n65 = Array Max & Min(array=w253) -> ()  [unwired: 4 out]
            n66 = To Unsigned Long Integer(number=w253) -> (unsigned 32bit integer=w258:u32[])
            n67 = Subtract(x=w258, y=100) -> (x-y=w257:u32[])
            n68 = Add Array Elements(numeric array=w257) -> (sum=w256:u32)
            n69 = Add(x=u32 2000, y=w256) -> (x+y=w251:u32)
          }
        }
      }
    }
    n70 = To Double Precision Float(number=w123) -> (double precision float=w121:dbl[][])
    n71 = To Double Precision Float(number=w122) -> (double precision float=w119:dbl[][])
    n72 = Array Max & Min(array=w119) -> (max value=w118:dbl)  [unwired: 3 out]
    "max value" <- w118
    n73 = Array Max & Min(array=w121) -> (max value=w120:dbl)  [unwired: 3 out]
    "max value 2" <- w120
    n74 = Max & Min(x=w120, y=w118) -> (max(x,y)=w117:dbl)  [unwired: 1 out]
    n75 = Divide(x=w119, y=w117) -> (x/y=w115:dbl[][])
    n76 = Compound Arithmetic op=MULTIPLY(w115, invert 1.0 ("y"), 255.0 ("value")) -> (w146:dbl[][])
    n77 = To Unsigned Byte Integer(number=w146) -> (unsigned 8bit integer=w113:u8[][])
    n78 = call "IMAQ ArrayToImage"("error in (no error)"=w141, "Image Pixels (U8)"=w113, "Image"=w144) -> ("error out"=w142:errorcluster, "Image Out"=w143:T4)  [unwired: 7 in]
    n79 = Divide(x=w121, y=w117) -> (x/y=w116:dbl[][])
    "Intensity Graph" <- w116
    n80 = Compound Arithmetic op=MULTIPLY(w116, invert 1.0 ("y"), 255.0 ("value")) -> (w149:dbl[][])
    n81 = To Unsigned Byte Integer(number=w149) -> (unsigned 8bit integer=w151:u8[][])
    n82 = call "IMAQ ArrayToImage"("error in (no error)"=w156, "Image Pixels (U8)"=w151, "Image"=w157) -> ("error out"=w155:errorcluster, "Image Out"=w140:T4)  [unwired: 7 in]
    "Image" <- w140
    n83 = case shown="False" w217 {
      tunnel: w140 -> [w313 w381]
      tunnel: w155 -> [w312 w393]
      tunnel: w213 -> [w311 w388]
      tunnel: [_ TRUE] -> w216
      tunnel: w214 -> [w315 _]
      tunnel: w209 -> [w314 w387]
      tunnel: [w310 w390] -> w134
      tunnel: [w309 w387] -> w212
      tunnel: [w308 w382] -> w124
      tunnel: [w307 w381] -> w135
      tunnel: "Max # of Matches" -> [w306 _]
      tunnel: "Minimum Score" -> [w305 _]
      tunnel: cluster{"Start Angle":sgl, "End Angle":sgl}[] [{"Start Angle"=0.0, "End Angle"=360.0}] ("Angle Ranges") -> [w304 _]
      tunnel: w143 -> [w303 _]
      tunnel: w142 -> [w302 _]
      tunnel: w139 -> [w301 w383]
      tunnel: w138 -> [w300 w384]
      tunnel: [w299 w384] -> w136
      tunnel: [w298 w383] -> w137
      tunnel: w114 -> [w297 _]
      tunnel: w114 -> [_ w380]
      tunnel: w113 -> [w296 _]
      frame False {
        n84 = case shown="True" w315 {
          tunnel: w314 -> [w320 w379]
          tunnel: w313 -> [w318 _]
          tunnel: w312 -> [w322 _]
          tunnel: w311 -> [w319 w357]
          tunnel: [w322 w377] -> w310
          tunnel: [w320 w379] -> w309
          tunnel: [w319 w357] -> w308
          tunnel: [w318 w363] -> w307
          tunnel: w306 -> [_ w371]
          tunnel: w305 -> [_ w370]
          tunnel: w304 -> [_ w368]
          tunnel: w303 -> [_ w367]
          tunnel: w302 -> [_ w366]
          tunnel: w301 -> [w317 w364]
          tunnel: w300 -> [w316 w365]
          tunnel: [w316 w360] -> w299
          tunnel: [w317 w359] -> w298
          tunnel: w297 -> [_ w358]
          tunnel: w296 -> [_ w347]
          frame False {
            n85 = Wait (ms)(milliseconds to wait=u32 10) -> ()  [unwired: 1 out]
          }
          frame True {
            n86 = local read "ROI"() -> (w348:T3)
            n87 = Unbundle(w348) -> ("Global Rectangle"=w353:i32[])  [unwired: 1 out]
            "Global Rectangle" <- w353
            n88 = Index Array(array=w353) -> (element #1=w334:i32, element #2=w332:i32, element #3=w335:i32, element #4=w333:i32)  [unwired: 4 in]
            n89 = Subtract(x=w335, y=w334) -> (x-y=w331:i32)
            n90 = Subtract(x=w333, y=w332) -> (x-y=w330:i32)
            n91 = call "IMAQ Clear Overlay"("error in (no error)"=w366, "Image"=w367) -> ("error out"=w376:errorcluster, "Image Out"=w373:T4)  [unwired: 8 in]
            n92 = Bundle("Max # of Matches"=w371, "Minimum Score"=w370, "Angle Ranges"=w368) -> (w369:T12)  [unwired: 1 in]
            n93 = Build Array(w331, w330) -> (w325:i32[])
            "appended array 3" <- w325
            n94 = Build Array(w334, w332, w335, w332, w335, w333, w334, w333) -> (w352:i32[])
            n95 = call "IMAQ Match Pattern 4"("Image"=w373, "Algorithm"=w358, "Template Image"=w357, "Parameters"=w369, "error in (no error)"=w376) -> ("Matches (pixel)"=w362:T2, "Number of Matches"=→"Number of Matches":i32, "error out"=w372:errorcluster)  [unwired: 6 in, 2 out]
            "Matches (pixel)" <- w362
            n96 = call "IMAQ ImageToArray"("Image"=w357) -> ("Image Pixels (U8)"=w324:u8[][])  [unwired: 3 in, 4 out]
            n97 = Array Size(array=w324) -> (size(s)=→"size(s)":i32[])
            n98 = Bundle By Name(cluster=T10 {"template"=[], "target img"=[], "image size"=[]}, "image size"=w325, "target img"=w347, "template"=w324) -> (w355:T10)
            n99 = call "Overlay Pattern Matching Results.vi"("error in"=w372, "Matches"=w362, "Image"=w373) -> ("error out"=w374:errorcluster, "Image Out"=w363:T4)  [unwired: 7 in]
            "Image 2" <- w363
            n100 = Index Array(array=w362) -> (element=w361:T13)  [unwired: 1 in]
            n101 = To Variant(anything=w355) -> (Variant=w354:variant)
            n102 = Unbundle By Name(w361) -> ("Bounding Box"=w356:cluster{"x":sgl, "y":sgl}[])
            n103 = vi-ref "projection transformation matching function.vi"() -> (w350:refnum<vi>)
            n104 = call-poly <vilib>:"Unconstrained Optimization.vi"("function data"=w354, "objective function"=w350, "stopping criteria"="stopping criteria", "start"=w352) -> ("number of function evaluations"=→"number of function evaluations":i32, "f(minimum)"=→"f(minimum)":dbl, "minimum"=w349:dbl[])  [unwired: 4 in, 1 out]
            "minimum" <- w349
            n105 = Index Array(array=w325) -> (element #1=w328:i32, element #2=w327:i32)  [unwired: 2 in]
            n106 = call <vilib>:"Simple Error Handler.vi"("error in (no error)"=w374) -> ("error out"=w378:errorcluster)  [unwired: 4 in, 4 out]
            n107 = Bundle By Name(cluster=T9 {"Interpolation Type"=enum."Bilinear", "Destination Width"=0, "Destination Height"=0, "Fill Value"=0.0} ("Options"), "Destination Width"=w328, "Destination Height"=w327) -> (w326:T9)
            n108 = call-poly "IMAQ Extract Tetragon"("error in (no error)"=w365, "Tetragon"=w356, "Image Dst"=w364, "Image Src"=w363) -> ("error out"=w360:errorcluster, "Image Dst Out"=w359:T4)  [unwired: 6 in]
            n109 = call <vilib>:"Clear Errors.vi"("error in (no error)"=w378) -> ("error out"=w377:errorcluster)  [unwired: 5 in, 1 out]
            n110 = call "tetragon extraction.vi"("Options"=w326, "target img"=w347, "X"=w349) -> ("Image Pixels (U8)"=w346:u8[][])  [unwired: 6 in, 2 out]
            n111 = To Word Integer(number=w324) -> (16bit integer=w343:i16[][])
            n112 = To Word Integer(number=w346) -> (16bit integer=w342:i16[][])
            n113 = Subtract(x=w342, y=w343) -> (x-y=w339:i16[][])
            "Intensity Graph 6" <- w339
            n114 = To Double Precision Float(number=w339) -> (double precision float=w341:dbl[][])
            n115 = Square(x=w341) -> (x^2=w338:dbl[][])
            n116 = Add Array Elements(numeric array=w338) -> (sum=w340:dbl)
            n117 = Square Root(x=w340) -> (sqrt(x)=→"sqrt(x)":dbl)
          }
        }
      }
      frame True {
        w394 = T14 {[], []}  # Clear ROI
        n118 = property on="Image" class="ImageControl"() -> ("ROI"=w396:T3)  [unwired: 2 in, 2 out]
        "ROI" <- w396
        n119 = Unbundle(w396) -> ("Global Rectangle"=w398:i32[])  [unwired: 1 out]
        n120 = call "IMAQ Extract 2"("Optional Rectangle"=w398, "error in (no error)"=w393, "Image Dst"=w388, "Image Src"=w381) -> ("error out"=w386:errorcluster, "Image Dst Out"=w397:T4)  [unwired: 6 in]
        n121 = call "IMAQ Learn Pattern 6"("Image"=w397, "Algorithm"=w380, "Angle Range"=cluster{"Start Angle":sgl, "End Angle":sgl} {"Start Angle"=0.0, "End Angle"=360.0}, "error in (no error)"=w386) -> ("Template Image Out"=w382:T4, "error out"=w389:errorcluster)  [unwired: 9 in, 1 out]
        n122 = property on="Image" class="ImageControl"(error in=w389, "ROI"=w394) -> (error out=w395:errorcluster)  [unwired: 1 in, 1 out]
        n123 = call <vilib>:"Simple Error Handler.vi"("error in (no error)"=w395) -> ("error out"=w391:errorcluster)  [unwired: 4 in, 4 out]
        n124 = call <vilib>:"Clear Errors.vi"("error in (no error)"=w391) -> ("error out"=w390:errorcluster)  [unwired: 5 in, 1 out]
      }
    }
    n125 = Array Size(array=w116) -> (size(s)=w180:i32[])
    n126 = property on="Intensity Graph" class="IntGraph (strict)"() -> ("XScale.Maximum"=w170:dbl, "XScale.Minimum"=w171:dbl, "YScale.Maximum"=w172:dbl, "YScale.Minimum"=w173:dbl)  [unwired: 2 in, 2 out]
    n127 = Negate(x="max 3") -> (-x=w126:dbl)
    n128 = Subtract(x="max", y="min") -> (x-y=w167:dbl)
    n129 = Index Array(array=w180) -> (element #2=w181:i32)  [unwired: 2 in, 1 out]
    n130 = Subtract(x="max 3", y=w126) -> (x-y=w128:dbl)
    n131 = for {
      N: 5 ("num of colors 3") -> [w227]
      tunnel: w128 -> [w231]
      tunnel: [w229] -> w112 mode=indexing
      tunnel: u32[] [0, 255, 16448250, 16711680, 16776960, 16711680, 16448250, 16448250] ("Array 4") -> [w228] mode=indexing
      tunnel: w126 -> [w223]
      i -> [w233]
      n132 = Decrement(x=w227) -> (x-1=w226:i32)
      n133 = Reciprocal(x=w226) -> (1/x=w225:dbl)
      n134 = Multiply(x=w225, y=w233) -> (x*y=w232:dbl)
      n135 = Multiply(x=w231, y=w232) -> (x*y=w230:dbl)
      n136 = Add(x=w223, y=w230) -> (x+y=w224:dbl)
      n137 = Bundle(w224, w228) -> (w229:cluster{dbl, u32})  [unwired: 1 in]
    }
    n138 = for {
      N: "num of colors" -> [w289]
      tunnel: w167 -> [w293]
      tunnel: [w291] -> w169 mode=indexing
      tunnel: "Array 2" -> [w290] mode=indexing
      tunnel: "min" -> [w285]
      i -> [w295]
      n139 = Decrement(x=w289) -> (x-1=w288:i32)
      n140 = Reciprocal(x=w288) -> (1/x=w287:dbl)
      n141 = Multiply(x=w287, y=w295) -> (x*y=w294:dbl)
      n142 = Multiply(x=w293, y=w294) -> (x*y=w292:dbl)
      n143 = Add(x=w285, y=w292) -> (x+y=w286:dbl)
      n144 = Bundle(w286, w290) -> (w291:cluster{dbl, u32})  [unwired: 1 in]
    }
    n145 = call "IMAQ ImageToArray"("error in (no error)"=w136, "Image"=w137) -> ("Image Pixels (U8)"=w133:u8[][])  [unwired: 2 in, 4 out]
    n146 = call "IMAQ ImageToArray"("error in (no error)"=w134, "Image"=w124) -> ("Image Pixels (U8)"=w125:u8[][])  [unwired: 2 in, 4 out]
    n147 = To Word Integer(number=w133) -> (16bit integer=w132:i16[][])
    n148 = To Word Integer(number=w125) -> (16bit integer=w131:i16[][])
    n149 = Subtract(x=w170, y=w171) -> (x-y=w177:dbl)
    n150 = Subtract(x=w172, y=w173) -> (x-y=w178:dbl)
    n151 = Multiply(x=w181, y="zoom") -> (x*y=w175:dbl)
    n152 = Divide(x=w177, y=w178) -> (x/y=w176:dbl)
    n153 = Subtract(x=w132, y=w131) -> (x-y=w107:i16[][])
    "Intensity Graph 5" <- w107
    n154 = Or(x=w134, y="Stop") -> (x .or. y?=w205:bool)
    n155 = Multiply(x=w175, y=w176) -> (x*y=w179:dbl)
    n156 = To Double Precision Float(number=w107) -> (double precision float=w108:dbl[][])
    n157 = property on="Intensity Graph" class="IntGraph (strict)"("Height"=w175, "Width"=w179) -> ()  [unwired: 2 in, 2 out]
    n158 = Square(x=w108) -> (x^2=w110:dbl[][])
    n159 = property on="Intensity Graph" class="IntGraph (strict)"("ZScale.MarkerVals[]"=w169) -> ()  [unwired: 2 in, 2 out]
    n160 = Add Array Elements(numeric array=w110) -> (sum=w109:dbl)
    n161 = property on="Intensity Graph 6" class="IntGraph (strict)"("ZScale.MarkerVals[]"=w112) -> ()  [unwired: 2 in, 2 out]
    n162 = property on="Intensity Graph 5" class="IntGraph (strict)"("ZScale.MarkerVals[]"=w112) -> ()  [unwired: 2 in, 2 out]
    n163 = Square Root(x=w109) -> (sqrt(x)=→"sqrt(x) 2":dbl)
  }
  n164 = Decrement(x=w13) -> (x-1=w9:i32)
  n165 = case shown="False" "skip matching" {
    tunnel: w66 -> [w436 _]
    tunnel: w65 -> [w435 _]
    tunnel: w64 -> [w434 _]
    tunnel: w63 -> [w433 _]
    tunnel: w62 -> [w432 _]
    tunnel: w61 -> [w431 _]
    tunnel: w60 -> [w430 _]
    tunnel: w59 -> [w421 w613]
    tunnel: w58 -> [w420 w612]
    tunnel: w56 -> [w405 w607]
    tunnel: [w404 w606] -> w42
    tunnel: [w403 w613] -> w38
    tunnel: [w402 w612] -> w1
    tunnel: w11 -> [w400 _]
    tunnel: w9 -> [w399 _]
    frame False {
      n166 = Set File Position(offset (in bytes) (0)=w400, refnum=w421, error in=w420) -> (refnum out=w423:refnum<file>, error out=w422:errorcluster)  [unwired: 1 in]
      n167 = Read from Binary File(5:u16[][][][] [], 8:w422, 11:w423) -> (0:w418:errorcluster, 2:w417:u16[][][][], 3:w419:refnum<file>)  [unwired: 3 in, 1 out]
      n168 = for {
        N: w399 -> [_]
        tunnel: w434 -> [w557]
        tunnel: w432 -> [w510]
        tunnel: w433 -> [w556]
        tunnel: [w540] -> w427
        tunnel: [w509] -> w425
        tunnel: [w506] -> w426
        tunnel: [w498] -> w402
        tunnel: [w499] -> w403
        tunnel: w418 -> [w500]
        tunnel: w419 -> [w501]
        tunnel: w431 -> [w548]
        tunnel: w430 -> [w545]
        tunnel: w436 -> [w544]
        tunnel: w435 -> [w543]
        tunnel: [w542] -> w429
        tunnel: [w541] -> w428
        shift-right: [w487] -> _
        shift-left: w417 -> [w496]
        tunnel: [w494] -> w410 mode=indexing
        tunnel: [w473] -> w412 mode=indexing
        tunnel: [w472] -> w408 mode=indexing
        tunnel: [w471] -> w409 mode=indexing
        tunnel: [w451] -> w407
        tunnel: [w440] -> w401
        i -> [w439]
        (unwired) TRUE
        w508 = 1 items=["All", "Low Discrepancy Sampling", "Grayscale Value Pyramid", "Gradients Pyramid"] ("Algorithm")
        n169 = Read from Binary File(5:u16[][][][] [], 8:w500, 11:w501) -> (0:w498:errorcluster, 2:w487:u16[][][][], 3:w499:refnum<file>)  [unwired: 3 in, 1 out]
        n170 = local read "channel"() -> (w495:i32)
        n171 = Index Array(array=w487, index (dim 0)=w495) -> (element=w562:u16[][][])  [unwired: 3 in]
        n172 = Index Array(array=w496, index (dim 0)=w495) -> (element=w566:u16[][][])  [unwired: 3 in]
        n173 = Array Size(array=w562) -> (size(s)=w559:i32[])
        n174 = Array Size(array=w566) -> (size(s)=w563:i32[])
        n175 = Index Array(array=w559) -> (element #2=w560:i32, element #3=w561:i32)  [unwired: 3 in, 1 out]
        n176 = Index Array(array=w563) -> (element #2=w564:i32, element #3=w565:i32)  [unwired: 3 in, 1 out]
        n177 = for {
          N: w560 -> [_]
          tunnel: w562 -> [w589]
          tunnel: [w587] -> w535 mode=indexing
          tunnel: w561 -> [w586]
          i -> [w588]
          n178 = for {
            N: w586 -> [_]
            tunnel: w589 -> [w600]
            tunnel: w588 -> [w599]
            tunnel: [w590] -> w587 mode=indexing
            i -> [w598]
            n179 = Index Array(array=w600, index (dim 1)=w599, index (dim 2)=w598) -> (element=w592:u16[])  [unwired: 1 in]
            n180 = for {
              tunnel: w592 -> [w603] mode=indexing
              tunnel: [w601] -> w591 mode=indexing
              n181 = Equal To 0?(x=w603) -> (x = 0?=w604:bool)
              n182 = Select(t=u16 100, s=w604, f=w603) -> (s? t:f=w601:u16)
            }
            n183 = Array Max & Min(array=w591) -> ()  [unwired: 4 out]
            n184 = To Unsigned Long Integer(number=w591) -> (unsigned 32bit integer=w597:u32[])
            n185 = Subtract(x=w597, y=100) -> (x-y=w596:u32[])
            n186 = Add Array Elements(numeric array=w596) -> (sum=w595:u32)
            n187 = Add(x=u32 2000, y=w595) -> (x+y=w590:u32)
          }
        }
        n188 = for {
          N: w564 -> [_]
          tunnel: w566 -> [w570]
          tunnel: w565 -> [w568]
          tunnel: [w567] -> w534 mode=indexing
          i -> [w569]
          n189 = for {
            N: w568 -> [_]
            tunnel: w570 -> [w581]
            tunnel: w569 -> [w580]
            tunnel: [w571] -> w567 mode=indexing
            i -> [w579]
            n190 = Index Array(array=w581, index (dim 1)=w580, index (dim 2)=w579) -> (element=w572:u16[])  [unwired: 1 in]
            n191 = for {
              tunnel: w572 -> [w584] mode=indexing
              tunnel: [w582] -> w573 mode=indexing
              n192 = Equal To 0?(x=w584) -> (x = 0?=w585:bool)
              n193 = Select(t=u16 100, s=w585, f=w584) -> (s? t:f=w582:u16)
            }
            n194 = Array Max & Min(array=w573) -> ()  [unwired: 4 out]
            n195 = To Unsigned Long Integer(number=w573) -> (unsigned 32bit integer=w578:u32[])
            n196 = Subtract(x=w578, y=100) -> (x-y=w577:u32[])
            n197 = Add Array Elements(numeric array=w577) -> (sum=w576:u32)
            n198 = Add(x=u32 2000, y=w576) -> (x+y=w571:u32)
          }
        }
        n199 = local read "Max # of Matches"() -> (w505:i32)
        n200 = local read "Minimum Score"() -> (w504:sgl)
        n201 = Bundle("Max # of Matches"=w505, "Minimum Score"=w504) -> ()  [unwired: 1 in, 1 out]
        n202 = Bundle("Max # of Matches"=w505, "Minimum Score"=w504, "Angle Ranges"=cluster{"Start Angle":sgl, "End Angle":sgl}[] [{"Start Angle"=0.0, "End Angle"=360.0}]) -> (w522:T12)  [unwired: 1 in]
        n203 = To Double Precision Float(number=w535) -> (double precision float=w533:dbl[][])
        n204 = To Double Precision Float(number=w534) -> (double precision float=w531:dbl[][])
        n205 = local read "stopping criteria"() -> (w453:T1)
        n206 = Array Max & Min(array=w531) -> (max value=w530:dbl)  [unwired: 3 out]
        n207 = Array Max & Min(array=w533) -> (max value=w532:dbl)  [unwired: 3 out]
        n208 = vi-ref "projection transformation matching function.vi"() -> (w461:refnum<vi>)
        n209 = Max & Min(x=w532, y=w530) -> (max(x,y)=w529:dbl)  [unwired: 1 out]
        n210 = Divide(x=w531, y=w529) -> (x/y=w488:dbl[][])
        n211 = Compound Arithmetic op=MULTIPLY(w488, invert 1.0 ("y"), 255.0 ("value")) -> (w550:dbl[][])
        n212 = To Unsigned Byte Integer(number=w550) -> (unsigned 8bit integer=w489:u8[][])
        n213 = call "IMAQ ArrayToImage"("error in (no error)"=w545, "Image Pixels (U8)"=w489, "Image"=w548) -> ("error out"=w546:errorcluster, "Image Out"=w547:T4)  [unwired: 7 in]
        n214 = call "IMAQ Clear Overlay"("error in (no error)"=w546, "Image"=w547) -> ("error out"=w525:errorcluster, "Image Out"=w524:T4)  [unwired: 8 in]
        n215 = Divide(x=w533, y=w529) -> (x/y=w503:dbl[][])
        n216 = Array Size(array=w503) -> (size(s)=w514:i32[])
        n217 = Compound Arithmetic op=MULTIPLY(w503, invert 1.0 ("y"), 255.0 ("value")) -> (w553:dbl[][])
        n218 = Multiply(x=w514, y=0.1) -> (x*y=w513:dbl[])
        n219 = Multiply(x=w514, y=0.9) -> (x*y=w512:dbl[])
        n220 = To Unsigned Byte Integer(number=w553) -> (unsigned 8bit integer=w555:u8[][])
        n221 = Index Array(array=w512) -> (element #1=w491:dbl, element #2=w490:dbl)  [unwired: 2 in]
        n222 = Index Array(array=w513) -> (element #1=w493:dbl, element #2=w492:dbl)  [unwired: 2 in]
        n223 = call "IMAQ ArrayToImage"("error in (no error)"=w556, "Image Pixels (U8)"=w555, "Image"=w557) -> ("error out"=w507:errorcluster, "Image Out"=w511:T4)  [unwired: 7 in]
        n224 = Build Array(w492, w493, w490, w491) -> (w470:dbl[])
        n225 = Round To Nearest(number=w470) -> (nearest integer value=w451:dbl[])
        "appended array" <- w451
        n226 = call "IMAQ Extract 2"("Optional Rectangle"=w451, "error in (no error)"=w507, "Image Dst"=w510, "Image Src"=w511) -> ("error out"=w518:errorcluster, "Image Dst Out"=w519:T4)  [unwired: 6 in]
        n227 = call "IMAQ Learn Pattern 6"("Image"=w519, "Algorithm"=w508, "Angle Range"=cluster{"Start Angle":sgl, "End Angle":sgl} {"Start Angle"=0.0, "End Angle"=360.0}, "error in (no error)"=w518) -> ("Template Image Out"=w509:T4)  [unwired: 9 in, 2 out]
        n228 = Index Array(array=w451) -> (element #1=w449:dbl, element #2=w447:dbl, element #3=w450:dbl, element #4=w448:dbl)  [unwired: 4 in]
        n229 = Subtract(x=w450, y=w449) -> (x-y=w446:dbl)
        n230 = Subtract(x=w448, y=w447) -> (x-y=w445:dbl)
        n231 = Build Array(w446, w445) -> (w440:dbl[])
        n232 = call "IMAQ Match Pattern 4"("Image"=w524, "Algorithm"=w508, "Template Image"=w509, "Parameters"=w522, "error in (no error)"=w525) -> ("Matches (pixel)"=w521:T2, "error out"=w523:errorcluster)  [unwired: 6 in, 3 out]
        n233 = Index Array(array=w451) -> (element #1=w464:dbl, element #2=w466:dbl, element #3=w465:dbl, element #4=w463:dbl)  [unwired: 4 in]
        n234 = call "IMAQ ImageToArray"("Image"=w509) -> ("Image Pixels (U8)"=w460:u8[][])  [unwired: 3 in, 4 out]
        n235 = Index Array(array=w521) -> (element=w520:T13)  [unwired: 1 in]
        n236 = Bundle By Name(cluster=T10 {"template"=[], "target img"=[], "image size"=[]}, "image size"=w440, "target img"=w489, "template"=w460) -> (w468:T10)
        n237 = Build Array(w464, w466, w465, w466, w465, w463, w464, w463) -> (w462:dbl[])
        n238 = Index Array(array=w440) -> (element #1=w444:dbl, element #2=w441:dbl)  [unwired: 2 in]
        n239 = Unbundle By Name(w520) -> ("Bounding Box"=w486:cluster{"x":sgl, "y":sgl}[])
        n240 = call "Overlay Pattern Matching Results.vi"("error in"=w523, "Matches"=w521, "Image"=w524) -> ("error out"=w506:errorcluster, "Image Out"=w540:T4)  [unwired: 7 in]
        n241 = Bundle By Name(cluster=T9 {"Interpolation Type"=enum."Bilinear", "Destination Width"=0, "Destination Height"=0, "Fill Value"=0.0} ("Options"), "Destination Width"=w444, "Destination Height"=w441) -> (w443:T9)
        n242 = To Variant(anything=w468) -> (Variant=w467:variant)
        n243 = call-poly <vilib>:"Unconstrained Optimization.vi"("function data"=w467, "objective function"=w461, "stopping criteria"=w453, "start"=w462) -> ("minimum"=w494:dbl[])  [unwired: 4 in, 3 out]
        "minimum 2" <- w494
        n244 = Index Array(array=w486) -> (element #1=w485:cluster{"x":sgl, "y":sgl}, element #2=w484:cluster{"x":sgl, "y":sgl}, element #3=w483:cluster{"x":sgl, "y":sgl}, element #4=w482:cluster{"x":sgl, "y":sgl})  [unwired: 4 in]
        n245 = call-poly "IMAQ Extract Tetragon"("error in (no error)"=w543, "Tetragon"=w486, "Image Dst"=w544, "Image Src"=w540) -> ("error out"=w541:errorcluster, "Image Dst Out"=w542:T4)  [unwired: 6 in]
        n246 = call "tetragon extraction.vi"("Options"=w443, "target img"=w489, "X"=w494) -> ("Image Pixels (U8)"=w459:u8[][])  [unwired: 6 in, 2 out]
        n247 = Unbundle(w485) -> ("x"=w481:sgl, "y"=w480:sgl)
        n248 = Unbundle(w484) -> ("x"=w479:sgl, "y"=w478:sgl)
        n249 = Unbundle(w483) -> ("x"=w477:sgl, "y"=w476:sgl)
        n250 = Unbundle(w482) -> ("x"=w475:sgl, "y"=w474:sgl)
        n251 = To Word Integer(number=w460) -> (16bit integer=w458:i16[][])
        n252 = To Word Integer(number=w459) -> (16bit integer=w457:i16[][])
        n253 = Build Array(w481, w480, w479, w478, w477, w476, w475, w474) -> (w473:sgl[])
        "appended array 2" <- w473
        n254 = call "IMAQ ImageToArray"("error in (no error)"=w541, "Image"=w542) -> ("Image Pixels (U8)"=w539:u8[][])  [unwired: 2 in, 4 out]
        n255 = call "IMAQ ImageToArray"("error in (no error)"=w506, "Image"=w509) -> ("Image Pixels (U8)"=w536:u8[][])  [unwired: 2 in, 4 out]
        n256 = Subtract(x=w457, y=w458) -> (x-y=w452:i16[][])
        n257 = local write "Intensity Graph"(w503) -> ()
        n258 = To Word Integer(number=w539) -> (16bit integer=w538:i16[][])
        n259 = To Word Integer(number=w536) -> (16bit integer=w537:i16[][])
        n260 = local write "Intensity Graph 6"(w452) -> ()
        n261 = To Double Precision Float(number=w452) -> (double precision float=w456:dbl[][])
        n262 = Subtract(x=w538, y=w537) -> (x-y=w502:i16[][])
        n263 = Square(x=w456) -> (x^2=w454:dbl[][])
        n264 = To Double Precision Float(number=w502) -> (double precision float=w526:dbl[][])
        n265 = Add Array Elements(numeric array=w454) -> (sum=w455:dbl)
        n266 = local write "Intensity Graph 5"(w502) -> ()
        n267 = Square Root(x=w455) -> (sqrt(x)=w472:dbl)
        "sqrt(x) 4" <- w472
        n268 = Square(x=w526) -> (x^2=w528:dbl[][])
        n269 = Add Array Elements(numeric array=w528) -> (sum=w527:dbl)
        n270 = Square Root(x=w527) -> (sqrt(x)=w471:dbl)
        "sqrt(x) 3" <- w471
        "Numeric" <- w439
      }
      n271 = Open/Create/Replace File(file path (use dialog)=w405, operation (0:open)=T5."replace or create") -> (refnum out=w416:refnum<file>, error out=w415:errorcluster)  [unwired: 4 in, 1 out]
      n272 = Bundle(cluster=T15 {"output tetragon rigid"=[], "output tetragon proj"=[], "error rigid"=[], "error proj"=[], "input rectangle"=[], "image size"=[]}, "output tetragon rigid"=w412, "output tetragon proj"=w410, "error rigid"=w409, "error proj"=w408, "input rectangle"=w407, "image size"=w401) -> (w404:T15)
      n273 = call "IMAQ Dispose"("Image"=w427, "error in (no error)"=w426) -> ("error out"=w438:errorcluster)  [unwired: 4 in]
      n274 = Write to Binary File(file (use dialog)=w416, data=w404, error in=w415) -> (refnum out=w413:refnum<file>, error out=w414:errorcluster)  [unwired: 3 in, 1 out]
      n275 = call "IMAQ Dispose"("Image"=w429, "error in (no error)"=w428) -> ()  [unwired: 4 in, 1 out]
      n276 = call "IMAQ Dispose"("Image"=w425, "error in (no error)"=w438) -> ("error out"=w437:errorcluster)  [unwired: 4 in]
      n277 = Close File(refnum=w413, error in=w414) -> ()  [unwired: 2 out]
      n278 = call <vilib>:"Simple Error Handler.vi"("error in (no error)"=w437) -> ()  [unwired: 4 in, 5 out]
    }
    frame True {
      n279 = Open/Create/Replace File(file path (use dialog)=w607) -> (refnum out=w608:refnum<file>, error out=w609:errorcluster)  [unwired: 5 in, 1 out]
      n280 = Read from Binary File(5:T15 {"output tetragon rigid"=[], "output tetragon proj"=[], "error rigid"=[], "error proj"=[], "input rectangle"=[], "image size"=[]}, 8:w609, 11:w608) -> (0:w610:errorcluster, 2:w606:T15, 3:w611:refnum<file>)  [unwired: 3 in, 1 out]
      n281 = Close File(refnum=w611, error in=w610) -> ()  [unwired: 2 out]
    }
  }
  n282 = Quotient & Remainder(x=w13, y="mabiki") -> (floor(x/y)=w5:i32)  [unwired: 1 out]
  n283 = Index Array(array=w14) -> (element #3=w12:i32, element #4=w2:i32, element #5=w3:i32)  [unwired: 5 in, 2 out]
  n284 = Replace Array Subset(array=w14, new element=w5, index=0) -> (w15:i32[])
  n285 = Unbundle By Name(w42) -> ("output tetragon proj"=w41:dbl[][], "input rectangle"=w40:dbl[])  [unwired: 4 out]
  n286 = Decrement(x=w2) -> (x-1=w6:i32)
  n287 = Decrement(x=w3) -> (x-1=w7:i32)
  n288 = Build Array(w7, w6) -> (w51:i32[])
  n289 = Build Array(w45, w6) -> (w50:dbl[])
  n290 = Build Array(w45, w45) -> (w55:dbl[])
  n291 = Build Array(w7, w45) -> (w52:dbl[])
  n292 = Build Array(w45, w45, w7, w45, w7, w6, w45, w6) -> (w44:dbl[])
  n293 = Open/Create/Replace File(file path (use dialog)=w18, error in=w1, operation (0:open)=T5."replace or create") -> (refnum out=w26:refnum<file>, error out=w25:errorcluster)  [unwired: 3 in, 1 out]
  n294 = Insert Into Array(array=w50, index=w53, new element=w54) -> (w49:dbl[])
  n295 = Insert Into Array(array=w51, index=w53, new element=w54) -> (w48:i32[])
  n296 = Insert Into Array(array=w52, index=w53, new element=w54) -> (w47:dbl[])
  n297 = Insert Into Array(array=w55, index=w53, new element=w54) -> (w46:dbl[])
  n298 = Write to Binary File(file (use dialog)=w26, data=w17, error in=w25) -> (refnum out=w28:refnum<file>, error out=w27:errorcluster)  [unwired: 3 in, 1 out]
  n299 = Write to Binary File(file (use dialog)=w28, data=w15, error in=w27) -> (refnum out=w30:refnum<file>, error out=w29:errorcluster)  [unwired: 3 in, 1 out]
  n300 = while {
    tunnel: w41 -> [w667]
    tunnel: w40 -> [w668]
    tunnel: w49 -> [w666]
    tunnel: w48 -> [w665]
    tunnel: w47 -> [w664]
    tunnel: w46 -> [w663]
    tunnel: w44 -> [w660]
    tunnel: "mabiki" -> [w655]
    tunnel: "mabiki" -> [w657]
    tunnel: w38 -> [w649]
    tunnel: w1 -> [w648]
    tunnel: [w647] -> w37
    tunnel: [w646] -> w36
    tunnel: w3 -> [w643]
    tunnel: [w637] -> w32
    tunnel: [w638] -> w31
    tunnel: w30 -> [w640]
    tunnel: w29 -> [w639]
    tunnel: w12 -> [w636]
    tunnel: w11 -> [w634]
    tunnel: w10 -> [w633]
    tunnel: w2 -> [w628]
    tunnel: w5 -> [w622]
    tunnel: "save transformed imgs" -> [w617]
    i -> [w616]
    stop <- w618 stop-if-true
    n301 = Decrement(x=w622) -> (x-1=w621:i32)
    n302 = Equal?(x=w621, y=w616) -> (x = y?=w620:bool)
    n303 = Select(t=w616, s=w617, f="review index") -> (s? t:f=w614:i32)
    n304 = Select(t=w620, s=w617, f="stop") -> (s? t:f=w618:bool)
    n305 = Multiply(x=w614, y=w657) -> (x*y=w631:i32)
    n306 = Multiply(x=w631, y=w633) -> (x*y=w635:i64)
    n307 = for {
      N: w655 -> [_]
      tunnel: w668 -> [w768]
      tunnel: w667 -> [w767]
      shift-right: [w742] -> _
      shift-left: _ -> [w763]
      tunnel: [w742] -> w623 mode=indexing
      tunnel: w666 -> [w746]
      tunnel: w665 -> [w745]
      tunnel: w664 -> [w744]
      tunnel: w663 -> [w743]
      tunnel: [w733] -> w662 mode=indexing
      tunnel: w631 -> [w731]
      i -> [w732]
      n308 = Add(x=w731, y=w732) -> (x+y=w730:i32)
      n309 = Index Array(array=w767, index (row)=w730) -> (element=w766:dbl[])  [unwired: 1 in]
      n310 = call "Projection transformation coefficients from rectangle input and output.vi"("output tetragon"=w766, "input rectangle"=w768) -> ("proj trans matrix"=w764:dbl[][])  [unwired: 1 out]
      n311 = Equal To 0?(x=w732) -> (x = 0?=w765:bool)
      n312 = case shown="False" w765 {
        tunnel: w764 -> [w770 w772]
        tunnel: [w769 w772] -> w742
        tunnel: w763 -> [w771 _]
        frame False {
          n313 = call-poly <vilib>:"A x B.vi"("B"=w771, "A"=w770) -> ("A x B"=w769:T16)  [unwired: 1 out]
        }
        frame True {
        }
      }
      n314 = call-poly <vilib>:"A x B.vi"("Vector"=w746, "A"=w742) -> ("A x Vector"=w762:dbl[])  [unwired: 1 out]
      n315 = call-poly <vilib>:"A x B.vi"("Vector"=w744, "A"=w742) -> ("A x Vector"=w754:dbl[])  [unwired: 1 out]
      n316 = call-poly <vilib>:"A x B.vi"("Vector"=w745, "A"=w742) -> ("A x Vector"=w755:dbl[])  [unwired: 1 out]
      n317 = call-poly <vilib>:"A x B.vi"("Vector"=w743, "A"=w742) -> ("A x Vector"=w747:dbl[])  [unwired: 1 out]
      n318 = Index Array(array=w762) -> (element #1=w761:dbl, element #2=w760:dbl, element #3=w759:dbl)  [unwired: 3 in]
      n319 = Index Array(array=w754) -> (element #1=w753:dbl, element #2=w752:dbl, element #3=w751:dbl)  [unwired: 3 in]
      n320 = Index Array(array=w755) -> (element #1=w756:dbl, element #2=w757:dbl, element #3=w758:dbl)  [unwired: 3 in]
      n321 = Index Array(array=w747) -> (element #1=w748:dbl, element #2=w749:dbl, element #3=w750:dbl)  [unwired: 3 in]
      n322 = Divide(x=w756, y=w758) -> (x/y=w737:dbl)
      n323 = Divide(x=w757, y=w758) -> (x/y=w736:dbl)
      n324 = Divide(x=w761, y=w759) -> (x/y=w735:dbl)
      n325 = Divide(x=w760, y=w759) -> (x/y=w734:dbl)
      n326 = Divide(x=w753, y=w751) -> (x/y=w739:dbl)
      n327 = Divide(x=w752, y=w751) -> (x/y=w738:dbl)
      n328 = Divide(x=w748, y=w750) -> (x/y=w741:dbl)
      n329 = Divide(x=w749, y=w750) -> (x/y=w740:dbl)
      n330 = Build Array(w741, w740, w739, w738, w737, w736, w735, w734) -> (w733:dbl[])
    }
    "A x B" <- w623
    n331 = Add(x=w635, y=w634) -> (x+y=w632:i64)
    n332 = Set File Position(offset (in bytes) (0)=w632, refnum=w649, error in=w648) -> (refnum out=w651:refnum<file>, error out=w652:errorcluster)  [unwired: 1 in]
    n333 = Read from Binary File(5:u16[][][][] [], 8:w652, 11:w651) -> (0:w646:errorcluster, 2:w645:u16[][][][], 3:w647:refnum<file>)  [unwired: 3 in, 1 out]
    n334 = Insert Into Array(array=w662, index (row)=0, new element=w660) -> (w659:dbl[][])  [unwired: 1 in]
    n335 = Increment(x=w655) -> (x+1=w656:i32)
    n336 = for {
      N: w636 -> [_]
      tunnel: [w722] -> w653 mode=indexing
      i -> [w723]
      n337 = Multiply(x=0.09, y=w723) -> (x*y=w722:dbl)
    }
    n338 = Transpose 2D Array(2D array=w659) -> (transposed array=w658:dbl[][])
    n339 = for {
      N: w656 -> [_]
      tunnel: [w724] -> w654 mode=indexing
      i -> [w724]
    }
    n340 = for {
      tunnel: w658 -> [w728] mode=indexing
      tunnel: [w727] -> w630 mode=indexing
      tunnel: w654 -> [w726]
      tunnel: w653 -> [w725]
      w729 = 3 items=["nearest", "linear", "spline", "cubic Hermite", "Lagrange"] ("method")
      n341 = call <vilib>:"Interpolate 1D.vi"("method"=w729, "xi"=w725, "X"=w726, "Y"=w728) -> ("yi"=w727:dbl[])  [unwired: 5 in, 2 out]
    }
    "Waveform Graph" <- w630
    n342 = Index Array(array=w645) -> (element #1=w627:u16[][][], element #2=w625:u16[][][])  [unwired: 8 in]
    n343 = for {
      tunnel: w625 -> [w670] mode=indexing
      tunnel: [w669] -> w624 mode=indexing
      n344 = for {
        tunnel: w670 -> [w672] mode=indexing
        tunnel: [w671] -> w669 mode=indexing
        n345 = for {
          tunnel: w672 -> [w675] mode=indexing
          tunnel: [w673] -> w671 mode=indexing
          n346 = Equal To 0?(x=w675) -> (x = 0?=w676:bool)
          n347 = Select(t=u16 100, s=w676, f=w675) -> (s? t:f=w673:u16)
        }
      }
    }
    n348 = for {
      tunnel: w627 -> [w678] mode=indexing
      tunnel: [w677] -> w626 mode=indexing
      n349 = for {
        tunnel: w678 -> [w680] mode=indexing
        tunnel: [w679] -> w677 mode=indexing
        n350 = for {
          tunnel: w680 -> [w683] mode=indexing
          tunnel: [w681] -> w679 mode=indexing
          n351 = Equal To 0?(x=w683) -> (x = 0?=w684:bool)
          n352 = Select(t=u16 100, s=w684, f=w683) -> (s? t:f=w681:u16)
        }
      }
    }
    n353 = Transpose 2D Array(2D array=w630) -> (transposed array=w644:dbl[][])
    n354 = for {
      tunnel: w626 -> [w714] mode=indexing
      tunnel: w624 -> [w713] mode=indexing
      tunnel: w644 -> [w719] mode=indexing
      tunnel: w643 -> [w716]
      tunnel: [w709] -> w629 mode=indexing
      tunnel: [w710] -> w642 mode=indexing
      tunnel: w628 -> [w715]
      w711 = T6 7 items=["Grayscale (U8)", "Grayscale (I16)", "Grayscale (SGL)", "Complex (CSG)", "RGB (U32)", "HSL (U32)", "RGB (U64)", "Grayscale (U16)"] ("Image Type")
      w712 = sgl 100.0 ("Fill Value")
      w718 = T9 {"Interpolation Type"=enum."Bilinear", "Destination Width"=0, "Destination Height"=0, "Fill Value"=0.0} ("Options")
      n355 = Bundle By Name(cluster=w718, "Destination Width"=w716, "Destination Height"=w715, "Fill Value"=w712) -> (w720:T9)
      n356 = Bundle By Name(cluster=w718, "Destination Width"=w716, "Destination Height"=w715, "Fill Value"=w712) -> (w717:T9)
      n357 = call "tetragon extraction.vi"("Options"=w717, "Image Type"=w711, "target img"=w713, "X"=w719) -> ("Image Pixels (U16)"=w710:u16[][])  [unwired: 5 in, 2 out]
      n358 = call "tetragon extraction.vi"("Options"=w720, "Image Type"=w711, "target img"=w714, "X"=w719) -> ("Image Pixels (U16)"=w709:u16[][])  [unwired: 5 in, 2 out]
    }
    n359 = Build Array(w629, w642) -> (w641:u16[][][][])
    n360 = while {
      tunnel: w629 -> [w696]
      tunnel: w626 -> [w695]
      tunnel: w617 -> [w685]
      stop <- w687 stop-if-true
      n361 = Array Size(array=w696) -> (size(s)=w697:i32[])
      n362 = Index Array(array=w697) -> (element #2=w698:i32, element #3=w699:i32)  [unwired: 3 in, 1 out]
      n363 = Index Array(array=w695, index (dim 0)="z index") -> (element=w693:u16[][])  [unwired: 2 in]
      "Intensity Graph 3" <- w693
      n364 = Index Array(array=w696, index (dim 0)="z index") -> (element=w692:u16[][])  [unwired: 2 in]
      "Intensity Graph 2" <- w692
      n365 = for {
        N: w698 -> [_]
        tunnel: w696 -> [w703]
        tunnel: [w701] -> _ mode=indexing
        tunnel: w699 -> [w700]
        i -> [w702]
        n366 = for {
          N: w700 -> [_]
          tunnel: w703 -> [w708]
          tunnel: w702 -> [w707]
          tunnel: [w705] -> w701 mode=indexing
          i -> [w706]
          n367 = Index Array(array=w708, index (dim 1)=w707, index (dim 2)=w706) -> (element=w704:u16[])  [unwired: 1 in]
          n368 = Array Max & Min(array=w704) -> (max value=w705:u16)  [unwired: 3 out]
        }
      }
      n369 = To Double Precision Float(number=w693) -> (double precision float=w690:dbl[][])
      n370 = To Double Precision Float(number=w692) -> (double precision float=w689:dbl[][])
      n371 = Subtract(x=w690, y=w689) -> (x-y=→"Intensity Graph 7":dbl[][])
      n372 = Select(t=TRUE, s=w685, f="quit review") -> (s? t:f=w687:bool)
    }
    n373 = Write to Binary File(file (use dialog)=w640, data=w641, error in=w639) -> (refnum out=w638:refnum<file>, error out=w637:errorcluster)  [unwired: 3 in, 1 out]
    "transform index" <- w616
  }
  n374 = Close File(refnum=w31, error in=w32) -> (error out=→"error out 2":errorcluster)  [unwired: 1 out]
  n375 = Close File(refnum=w37, error in=w36) -> (error out=→"error out":errorcluster)  [unwired: 1 out]
